vi "Main.vi"(11 "Module Admin":refnum<class "Delacor_lib_QMH_Module Admin.lvclass">) -> ()   [LabVIEW 2025, in "Scripting Server.lvlib"]
doc: "This template is based off of the Queued Message Handler design pattern and the Queued Message Handler project template that ships with LabVIEW.\n\nThe main difference is that the queue is private to this module and communication between modules is performed via Broadcast and Request events.\n\nRequest events are wrapped in public API methods and are handled in the Event Handling Loop (EHL) of this VI. Any module can register for Broadcast events sent by this module. The EHL generates messages based on user interface actions.\n\nThe Message Handling Loop (MHL) processes messages generated by the EHL, or by other messages. The messages are string values, so new messages can be added easily to the Message Cases case structure in the MHL. Each message cluster can also provide an optional value for Message Data, which is a variant that can be converted to whatever message-specific data is required.\n_____\nBased on DQMH Dev Tools: Project Template 7.1.0.1503."
uses:
  Scripting Server.lvlib
  <vilib>/Delacor/Delacor QMH/Libraries/Message Queue_class/Delacor_lib_QMH_Message Queue.lvclass/Delacor_lib_QMH_Message Queue.ctl
  <vilib>/Delacor/Delacor QMH/Libraries/Module Admin_class/Delacor_lib_QMH_Module Admin.lvclass/Delacor_lib_QMH_Module Admin.ctl
  <vilib>/Delacor/Delacor QMH/Libraries/Message Queue_class/Delacor_lib_QMH_Message Queue.lvclass
  Module Data--cluster.ctl
  <vilib>/Utility/miscctls.llb/LVPointTypeDef.ctl
  <vilib>/Delacor/Delacor QMH/Libraries/Message Queue_class/Delacor_lib_QMH_Enqueue Message (Single).vi
  Stop Argument--cluster.ctl
  <vilib>/Delacor/Delacor QMH/Libraries/Module Admin_class/Delacor_lib_QMH_Module Admin.lvclass
  New VI (Reply Payload)--cluster.ctl
  New VI Argument--cluster.ctl
  Add Object Argument--cluster.ctl
  Add Object (Reply Payload)--cluster.ctl
  Connect Objects (Reply Payload)--cluster.ctl
  Connect Objects Argument--cluster.ctl
  Get Object Terminals (Reply Payload)--cluster.ctl
  Get Object Terminals Argument--cluster.ctl
  get vi error list (Reply Payload)--cluster.ctl
  get vi error list Argument--cluster.ctl
  Cleanup VI (Reply Payload)--cluster.ctl
  Cleanup VI Argument--cluster.ctl
  create_control (Reply Payload)--cluster.ctl
  create_control Argument--cluster.ctl
  Run VI (Reply Payload)--cluster.ctl
  Run VI Argument--cluster.ctl
  add_to_selection (Reply Payload)--cluster.ctl
  add_to_selection Argument--cluster.ctl
  clear_selection_list (Reply Payload)--cluster.ctl
  clear_selection_list Argument--cluster.ctl
  remove_from_selection (Reply Payload)--cluster.ctl
  remove_from_selection Argument--cluster.ctl
  enclose_selection (Reply Payload)--cluster.ctl
  enclose_selection Argument--cluster.ctl
  rename_object (Reply Payload)--cluster.ctl
  rename_object Argument--cluster.ctl
  set_value (Reply Payload)--cluster.ctl
  set_value Argument--cluster.ctl
  delete_object (Reply Payload)--cluster.ctl
  delete_object Argument--cluster.ctl
  save_vi (Reply Payload)--cluster.ctl
  save_vi Argument--cluster.ctl
  get_structure_diagram (Reply Payload)--cluster.ctl
  get_structure_diagram Argument--cluster.ctl
  add_subvi (Reply Payload)--cluster.ctl
  add_subvi Argument--cluster.ctl
  connect_to_pane (Reply Payload)--cluster.ctl
  connect_to_pane Argument--cluster.ctl
  get_object_help (Reply Payload)--cluster.ctl
  get_object_help Argument--cluster.ctl
  get_loop_conditional_terminal (Reply Payload)--cluster.ctl
  get_loop_conditional_terminal Argument--cluster.ctl
  show_conditional_terminal (Reply Payload)--cluster.ctl
  show_conditional_terminal Argument--cluster.ctl
  get_loop_iteration_terminal (Reply Payload)--cluster.ctl
  get_loop_iteration_terminal Argument--cluster.ctl
  Config Data.ctl
  Read Config Data Argument--cluster.ctl
  get_allowed_paths (Reply Payload)--cluster.ctl
  get_allowed_paths Argument--cluster.ctl
  create_project (Reply Payload)--cluster.ctl
  create_project Argument--cluster.ctl
  Set Allowed Paths Argument--cluster.ctl
panel:
  in  "Ring 2":i32(ring)=2125 items=[".NET Container"=2125, ".NET Refnum"=3441, "2D Picture"=3508, "3D Picture"=23776, "Absolute Value"=1054, "Accept TLS"=1732, "Access Rights"=1412, "ActiveX Container"=2072, "Add"=1050, "Add (with error terminals)"=3915, "Add Array Elements"=1903, "Add Entropy"=1738, "Add Private Key To TLS Configuration"=1735, "Add Trusted Certificate To TLS Configuration"=1736, "Agitator"=3831, "AllSpoll"=1960, "Always Copy"=2400, "And"=1061, "And Array Elements"=1911, "Append True/False String"=1511, "Application Refnum"=3412, "Array (block diagram constant)"=2070, "Array (classic)"=3300, "Array (modern)"=21608, "Array Interface Control"=23777, "Array Max & Min"=1907, "Array of Strings to Path"=1422, "Array Size"=1809, "Array Subset"=2044, "Array To Cluster"=1168, "Array To Spreadsheet String"=1540, "ArrayMemInfo"=2412, "Assert Structural Type Match"=2416, "Assert Structural Type Mismatch"=2464, "Atmospheric Tank (classic)"=3070, "Atmospheric Tank (modern)"=21751, "Automation Close"=8001, "Automation Open"=8000, "Automation Refnum"=3410, "Avogadro Constant (1/mol)"=23520, "Base 10 Logarithm Of e"=23512, "Bin #1"=3073, "Bin #2"=21755, "Bitpack to Array"=3135, "Bluetooth Close Connection"=9148, "Bluetooth Create Listener"=9151, "Bluetooth Discover"=9152, "Bluetooth Network Connection Refnum"=3468, "Bluetooth Open Connection"=9153, "Bluetooth Read"=9149, "Bluetooth Wait On Listener"=9147, "Bluetooth Write"=9150, "Boolean Array To Number"=1815, "Boolean To (0,1)"=1167, "Build Array"=2041, "Build Cluster Array"=2047, "Build Map"=2463, "Build Matrix"=8500, "Build Path"=1419, "Build Set"=2462, "Build Waveform"=2066, "Bundle"=2049, "Bundle By Name"=2057, "Byte Array To String"=1609, "Byte Array To UTF-8 String"=1651, "Byte Stream File Refnum"=3408, "Call By Reference"=3901, "Call Chain"=1999, "Call Library Function Node"=2062, "Call MATLAB Function"=24210, "Call Parent Class Method"=2354, "CAN Channel (block diagram constant)"=2124, "CAN Channel (classic)"=3340, "CAN Channel (modern)"=21817, "CAN Channel (system)"=21966, "CAN Interface (block diagram constant)"=2123, "CAN Interface (classic)"=3339, "CAN Interface (modern)"=21815, "CAN Interface (system)"=21964, "CAN Task (block diagram constant)"=3471, "CAN Task (classic)"=3470, "CAN Task (modern)"=21789, "CAN Task (system)"=21963, "Cancel Button (modern)"=21739, "Cancel Button (system)"=3131, "Cancel Notification"=9107, "Carriage Return Constant"=23500, "Case Structure"=2001, "Cast Unit Bases"=1079, "Check Valve"=3833, "Checkbox (classic)"=3117, "CheckBox (modern)"=21924, "Checkbox (system)"=3132, "Class Specifier Constant"=2094, "Classic Color Box"=3013, "Classic Color Ramp"=3022, "Classic Horizontal Slide Switch"=3114, "Classic Vertical Slide"=3004, "Clear Fixed-Point Overflow Status"=5562, "Close File"=8052, "Close File (deprecated)"=1405, "Close MATLAB Session"=24209, "Close Python Session"=24207, "Close Reference"=8011, "Close TLS Configuration"=1741, "Close Variable Connection"=23783, "Closure Structure"=2372, "Cluster (classic)"=3400, "Cluster (modern)"=21607, "Cluster Constant"=2071, "Cluster To Array"=1169, "Code Interface Node"=2050, "Coerce To Type"=2402, "Collection Size"=2450, "Color Box Constant"=2120, "Color Box Thin Border"=2905, "Colored Rectangle (broken?)"=3625, "Combo Box (classic)"=3304, "Combo Box (modern)"=21604, "Combo Box (system)"=21917, "Combo Box Constant"=2088, "Complex Conjugate"=1048, "Complex To Polar"=1045, "Complex To Re/Im"=1044, "Compound Arithmetic"=2200, "Compressor"=3832, "Concatenate Strings"=2040, "Conditional Disable Structure"=2064, "Constructor Node"=3904, "Control & Simulation Loop"=2099, "Control Help Window"=1353, "Control Online Help"=1355, "Control Refnum"=3419, "Convert Unit"=2059, "Conveyer"=3827, "Copy"=8053, "Copy (deprecated)"=1416, "Cosecant"=1204, "Cosine"=1201, "Cotangent"=1205, "CPU Information"=24130, "Create Folder"=8055, "Create Network Stream Endpoint"=23793, "Create Network Stream Reader Endpoint"=23811, "Create Network Stream Writer Endpoint"=23810, "Create Stream"=23796, "Create Unique Network Stream Endpoint"=23795, "Create Unique Network Stream Reader Endpoint"=23807, "Create Unique Network Stream Writer Endpoint"=23806, "Create User Event"=2073, "Current Processor ID"=24131, "Current VI's Menubar"=9000, "Current VI's Path"=1426, "DAQmx Analog Trigger Source (block diagram constant)"=2119, "DAQmx Analog Trigger Source (classic)"=3336, "DAQmx Analog Trigger Source (modern)"=21774, "DAQmx Analog Trigger Source (system)"=21951, "DAQmx Device Name (block diagram constant)"=2093, "DAQmx Device Name (classic)"=3318, "DAQmx Device Name (modern)"=21773, "DAQmx Device Name (system)"=21950, "DAQmx Global Channel (block diagram constant)"=3430, "DAQmx Global Channel (classic)"=3443, "DAQmx Global Channel (modern)"=21770, "DAQmx Global Channel (system)"=21957, "DAQmx Physical Channel (block diagram constant)"=2118, "DAQmx Physical Channel (classic)"=3335, "DAQmx Physical Channel (modern)"=21777, "DAQmx Physical Channel (system)"=21954, "DAQmx Scale Name (block diagram constant)"=2116, "DAQmx Scale Name (classic)"=3317, "DAQmx Scale Name (modern)"=21775, "DAQmx Scale Name (system)"=21952, "DAQmx Switch (block diagram constant)"=2121, "DAQmx Switch (classic)"=3337, "DAQmx Switch (modern)"=21776, "DAQmx Switch (system)"=21953, "DAQmx Task Name (block diagram constant)"=3434, "DAQmx Task Name (classic)"=3442, "DAQmx Task Name (modern)"=21778, "DAQmx Task Name (system)"=21959, "DAQmx Terminal (block diagram constant)"=2117, "DAQmx Terminal (classic)"=3319, "DAQmx Terminal (modern)"=21781, "DAQmx Terminal (system)"=21955, "Data Cache Size"=24132, "Data Log File Refnum"=3402, "Data Value Reference"=3476, "Data Value Reference Constant"=24134, "DataSocket Close"=1085, "DataSocket Open"=1084, "DataSocket Read"=1086, "DataSocket Refnum"=3417, "DataSocket Write"=1087, "Date/Time To Seconds"=1308, "Decimal Digit?"=1119, "Decimal String To Number"=1184, "Decimate 1D Array"=2046, "DecomposeLockDataValRef"=2406, "DecomposeVariant"=2404, "Decrement"=1058, "Default Directory"=1427, "Delete"=8056, "Delete (deprecated)"=1417, "Delete Data Value Reference"=2409, "Delete From Array"=3912, "Delete Menu Items"=9004, "Delete Variant Attribute"=8206, "Delete Waveform Attribute"=8209, "Deny Access"=8057, "Dequeue Element"=9113, "Destroy Stream Endpoint"=23794, "Destroy User Event"=2075, "DevClear"=1961, "DevClearList"=1962, "Device Control/Status"=1433, "Device Refnum"=3405, "Diagram Disable Structure"=2054, "Dial (classic)"=3050, "Dial (modern)"=21732, "Digital Data (classic)"=3210, "Digital Data (modern)"=21216, "Digital Waveform Graph (classic)"=3511, "Digital Waveform Graph (modern)"=21718, "Direct Variable Read"=23785, "Direct Variable Write"=23788, "Divide"=1053, "Divide (with error terminals)"=3918, "Dlg Horiz Scrollbar"=21905, "Dlg Mac Group Box"=32514, "Dlg Numeric #1"=2100, "Dlg Numeric #2"=3006, "Dlg String"=2110, "Dlg Vert Scrollbar"=21906, "Down Arrow"=3824, "Down Bow Valve (flat)"=3707, "Down Bow Valve (outline)"=3807, "Down Bow Valve (shaded)"=21767, "Down Rect Valve (flat)"=3706, "Down Rect Valve (outline)"=3806, "Down Rect Valve (shaded)"=21766, "Down Tee (flat)"=3818, "Down Tee (shaded)"=3718, "Dynamic FPGA Interface Cast"=5690, "Eased Corner Rectangle"=32513, "Element of Set?"=2454, "Elementary Charge (C)"=23517, "Empty Array?"=23063, "Empty Collection?"=2451, "Empty Path Constant"=23523, "Empty String Constant"=23503, "Empty String/Path?"=1112, "Enable Menu Tracking"=9002, "EnableLocal"=1963, "EnableRemote"=1964, "End of Line Constant"=23525, "Enqueue Element"=9111, "Enqueue Element At Opposite End"=9129, "Enum (classic)"=3023, "Enum (modern)"=21605, "Enum (system)"=3062, "Enum Constant"=2090, "EOF"=1410, "Equal To 0?"=1113, "Equal?"=1102, "Error Ring Constant"=2039, "Event Callback Refnum"=3435, "Event Data Node"=2102, "Event Structure"=2052, "Exchanger"=3828, "Exclusive Or"=1063, "Exponential"=1211, "Exponential (Arg) -1"=1222, "Expression Node"=2201, "False Constant"=2006, "Feedback Node"=2353, "FieldPoint IO Point (block diagram constant)"=3440, "FieldPoint IO Point (classic)"=3439, "FieldPoint IO Point (modern)"=21784, "FIFO Refnum"=3474, "File Dialog"=8058, "File Dialog (deprecated)"=8081, "File Path Control (classic)"=3203, "File Path Control (modern)"=21730, "File Path Control (system)"=21922, "File Path Indicator (classic)"=3204, "File Path Indicator (modern)"=21731, "File/Directory Info"=8082, "File/Directory Info (deprecated)"=1413, "FindLstn"=1965, "FindRQS"=1966, "First Call?"=1083, "Fixed-Point Overflow?"=5565, "Fixed-Point to Integer Cast"=5566, "Flat Box"=3602, "Flat Circle"=3605, "Flat Down Triangle"=3623, "Flat Frame"=3608, "Flat Left Triangle"=3620, "Flat Right Triangle"=3621, "Flat Round Button"=3102, "Flat Rounded Box"=3611, "Flat Sequence Structure"=2069, "Flat Square Button"=3103, "Flat Up Triangle"=3622, "Flatten To JSON"=24201, "Flatten To String"=1164, "Flatten To XML"=8402, "Flattened String To Variant"=8202, "Floating Point Equal?"=23064, "Flush Event Queue"=2135, "Flush File"=8059, "Flush File (deprecated)"=1406, "Flush Queue"=9114, "Flush Stream"=23808, "For Loop"=2002, "Fork"=2194, "Format Date/Time String"=8100, "Format Into File"=2083, "Format Into String"=2081, "Format Value"=1512, "Formula Node"=2004, "FPGA Refnum to Session"=2322, "Fract/Exp String To Number"=1187, "Framed Color Box (classic)"=3008, "Framed Color Box (modern)"=21019, "Free Label"=2321, "Furnace"=3829, "Gauge (classic)"=3040, "Gauge (modern)"=21009, "Gauge for Simon"=32600, "Generate Front Panel Activity"=1329, "Generate Occurrence"=1700, "Generate User Event"=2074, "Generate User-Defined Trace Event"=2250, "Get Control Values by Index"=24204, "Get Datalog Position"=8061, "Get Date/Time In Seconds"=1303, "Get Date/Time String"=1600, "Get Drag Drop Data"=9154, "Get File Position"=8062, "Get File Size"=8063, "Get Fixed-Point Components"=11163, "Get Help Window Status"=1354, "Get Matrix Diagonal"=8501, "Get Matrix Elements"=8502, "Get Menu Item Info"=9005, "Get Menu Selection"=9001, "Get Menu Short Cut Info"=9007, "Get Notifier Status"=9103, "Get Number of Records"=8064, "Get Permissions"=8065, "Get Queue Status"=9110, "Get Submatrix"=8503, "Get Type and Creator"=8066, "Get Variant Attribute"=8205, "Get Volume Info"=8067, "Get Waveform Attribute"=8208, "Get Waveform Components"=2067, "Global Variable"=2060, "GPIB Clear"=1954, "GPIB Initialization"=1957, "GPIB Misc"=1956, "GPIB Read"=1951, "GPIB Serial Poll"=1955, "GPIB Status"=1959, "GPIB Trigger"=1953, "GPIB Wait"=1958, "GPIB Write"=1950, "Gravitational Constant (N m2/kg2)"=23519, "Greater Or Equal To 0?"=1114, "Greater Or Equal?"=1103, "Greater Than 0?"=1117, "Greater?"=1110, "Handle Peek"=1604, "Handle Poke"=1605, "Hex Digit?"=1123, "Hexadecimal String To Number"=1185, "Hopper #1"=21754, "Hopper #2"=3072, "Horiz Line"=3821, "Horiz Pipe (flat)"=3810, "Horiz Pipe (shaded)"=3710, "Horizontal Button Box"=3636, "Horizontal Fill Slide (classic)"=3012, "Horizontal Fill Slide (modern)"=21100, "Horizontal Gradient Oval"=32502, "Horizontal Gradient Rectangle"=32504, "Horizontal Gradient Rounded Rectangle"=32507, "Horizontal Graduated Bar"=21106, "Horizontal Pointer Slide (classic)"=3011, "Horizontal Pointer Slide (modern)"=21101, "Horizontal Pointer Slide (system)"=21902, "Horizontal Progress Bar (modern)"=21102, "Horizontal Progress Bar (system)"=21910, "Horizontal Scrollbar"=21110, "Horizontal Slide (classic)"=3010, "Horizontal Slide (system)"=21904, "Horizontal Smooth Box"=3633, "Horizontal Splitter Bar"=21861, "Horizontal Splitter Bar (Classic)"=21863, "Horizontal Splitter Bar (NXG Style)"=21867, "Horizontal Splitter Bar (System)"=21865, "Horizontal Switch"=3108, "Horizontal Tank"=3071, "Horizontal Toggle Switch (classic)"=3110, "Horizontal Toggle Switch (modern)"=21700, "Hyperbolic Cosecant"=23053, "Hyperbolic Cosine"=1215, "Hyperbolic Cotangent"=23055, "Hyperbolic Secant"=23054, "Hyperbolic Sine"=1214, "Hyperbolic Tangent"=1216, "IMAQ Session"=3415, "Implies"=1080, "In Place Element Structure"=2360, "In Range and Coerce"=1127, "Include Fixed-Point Overflow Status"=5564, "Increment"=1057, "Index & Bundle Cluster Array"=2056, "Index Array"=2042, "Index String Array"=1531, "Initialize Array"=2053, "Inline C Node"=2104, "Insert Into Array"=3911, "Insert Into Map"=2456, "Insert Into Set"=2452, "Insert Menu Items"=9003, "Integer to Fixed-Point Cast"=5567, "Intensity Chart (classic)"=3509, "Intensity Chart (modern)"=21719, "Intensity Graph (classic)"=3510, "Intensity Graph (modern)"=21720, "Interleave 1D Arrays"=2045, "Interpolate 1D Array"=1905, "Inverse Cosecant"=23050, "Inverse Cosine"=1207, "Inverse Cotangent"=23052, "Inverse Hyperbolic Cosecant"=23056, "Inverse Hyperbolic Cosine"=1218, "Inverse Hyperbolic Cotangent"=23058, "Inverse Hyperbolic Secant"=23057, "Inverse Hyperbolic Sine"=1217, "Inverse Hyperbolic Tangent"=1219, "Inverse Secant"=23051, "Inverse Sine"=1206, "Inverse Tangent"=1208, "Inverse Tangent (2 Input)"=1228, "Invoke Node"=3900, "IP To String"=1710, "IrDA Close Connection"=9144, "IrDA Create Listener"=9140, "IrDA Discover"=9141, "IrDA Network Connection Refnum"=3450, "IrDA Open Connection"=9142, "IrDA Read"=9145, "IrDA Wait On Listener"=9143, "IrDA Write"=9146, "IsDebuggingActive"=2403, "IVI Delete Session"=8103, "IVI Logical Name (block diagram constant)"=3420, "IVI Logical Name (classic)"=3414, "IVI Logical Name (modern)"=21736, "IVI New Session"=8102, "Join"=2195, "Join Numbers"=1171, "Junction"=2197, "Knob (classic)"=3005, "Knob (modern)"=21000, "Label (modern)"=21960, "Label (system)"=21961, "Labeled Oblong Button"=3125, "Labeled Rectangular Button"=3124, "Labeled Round Button"=3122, "Labeled Square Button"=3123, "LabVIEW Object"=3457, "Leak Variant Value Reference"=2410, "LED Button"=3116, "Left Arrow"=3826, "Left Bow Valve (flat)"=3701, "Left Bow Valve (outline)"=3801, "Left Bow Valve (shaded)"=21761, "Left Down Elbow (flat)"=3811, "Left Down Elbow (shaded)"=3711, "Left Pump (flat)"=3813, "Left Pump (shaded)"=3713, "Left Rect Valve (flat)"=3700, "Left Rect Valve (outline)"=3800, "Left Rect Valve (shaded)"=21760, "Left Tee (flat)"=3809, "Left Tee (shaded)"=3709, "Left Up Elbow (flat)"=3808, "Left Up Elbow (shaded)"=3708, "Less Or Equal To 0?"=1115, "Less Or Equal?"=1104, "Less Than 0?"=1118, "Less?"=1111, "Lexical Class"=1126, "Line (chiseled, system)"=3632, "Line (chiseled, thick)"=3630, "Line (chiseled, thin)"=3627, "Line (thick)"=3629, "Line (thin)"=3626, "Line Feed Constant"=23501, "Line with Arrow (thick)"=3631, "Line with Arrow (thin)"=3628, "List Directory"=1418, "List Folder"=8083, "Listbox (classic)"=21806, "Listbox (modern)"=21792, "Listbox (system)"=21805, "Listbox Symbol Ring Constant"=2038, "Load Certificates Into Memory"=1734, "Load Private Key Into Memory"=1733, "Local Variable"=2061, "Lock Range"=1411, "Logarithm Base 10"=1210, "Logarithm Base 2"=1225, "Logarithm Base X"=1224, "Logical Shift"=1081, "Look In Map"=2458, "Lookup Channel Probe"=9155, "Lossy Enqueue Element"=9130, "Lowered Box (thick)"=3635, "Lowered Rounded Box"=3638, "Machine Epsilon"=23528, "Make TLS Configuration Immutable"=1737, "MakeAddr"=1967, "Mantissa & Exponent"=1150, "Map"=3488, "Map Constant"=2461, "Match First String"=1532, "Match Pattern"=1535, "Match True/False String"=1533, "MathScript Call By Reference"=3906, "MathScript Node"=2357, "MATLAB script"=9020, "MATLAB Session Refnum"=3490, "Matrix Size"=8507, "Max & Min"=1108, "Menu Refnum"=3413, "Menu Ring (classic)"=3018, "Menu Ring (modern)"=21600, "Menu-Popup Ring"=3017, "Merge Errors"=2147, "Merge Signals"=2350, "Meter (classic)"=3030, "Meter (modern)"=21008, "Mixed Checkbox (system)"=21333, "Mixed Signal Graph"=21721, "Molar Gas Constant (J/(mol K))"=23522, "Motion Resource (block diagram constant)"=3449, "Motion Resource (classic)"=3448, "Motion Resource (modern)"=21787, "Motor (flat)"=3820, "Motor (shaded)"=3720, "Move"=8068, "Move (deprecated)"=1415, "Multi-Segment Pipe"=23780, "Multicolumn Listbox (classic)"=21799, "Multicolumn Listbox (modern)"=21791, "Multicolumn Listbox (system)"=21798, "Multiply"=1052, "Multiply (with error terminals)"=3917, "Multiply Array Elements"=1904, "Multirate Structure"=2199, "Natural Logarithm"=1209, "Natural Logarithm (Arg +1)"=1221, "Natural Logarithm Base"=23510, "Natural Logarithm Of 10"=23513, "Natural Logarithm Of 2"=23514, "Natural Logarithm Of Pi"=23508, "Negate"=1069, "Negative Infinity"=23509, "New Data Value Reference"=2408, "New Directory"=1402, "New File"=1404, "New TLS Configuration"=1730, "New VI"=8014, "New VI Object"=8015, "Not"=1064, "Not A Number/Path/Refnum?"=1128, "Not A Path Constant"=23524, "Not a Refnum Constant"=23526, "Not a Shared Variable"=23527, "Not And"=1071, "Not Equal To 0?"=1116, "Not Equal?"=1105, "Not Exclusive Or"=1073, "Not Or"=1072, "Notifier Refnum"=3423, "Number of Cache Levels"=24133, "Number To Boolean Array"=1814, "Number To Decimal String"=1180, "Number To Engineering String"=1183, "Number To Exponential String"=1505, "Number To Fractional String"=1506, "Number To Hexadecimal String"=1181, "Number To Octal String"=1182, "Numeric Constant"=2005, "Numeric Control (classic)"=3000, "Numeric Control (modern)"=21003, "Numeric Control (system)"=21919, "Numeric Indicator (classic)"=3001, "Numeric Indicator (modern)"=21004, "Obtain Notifier"=9101, "Obtain Queue"=9108, "Occurrence Refnum"=3406, "Octal Digit?"=1129, "Octal String To Number"=1186, "OK Button (modern)"=21738, "OK Button (system)"=3130, "Old VISA Open"=1921, "OLE Variant"=3150, "One Button Dialog"=1340, "Open and Verify Variable Connection"=23790, "Open Application Reference"=8012, "Open Device"=1430, "Open Dynamic Bitfile Reference"=5691, "Open File"=1403, "Open MATLAB Session"=24208, "Open Python Session"=24206, "Open Tank (flat classic)"=21752, "Open Tank (shaded classic)"=3074, "Open Variable Connection"=23779, "Open Variable Connection in Background"=23791, "Open VI Object Reference"=8013, "Open VI Reference"=8010, "Open/Create/Replace Datalog"=8054, "Open/Create/Replace File"=8050, "Or"=1062, "Or Array Elements"=1910, "Oval with Shadow"=32509, "Package Matrix"=23001, "PassControl"=1968, "Path Constant"=2009, "Path to Array of Strings"=1423, "Path To String"=1077, "Path Type"=1421, "Pi"=23504, "Pi Divided By 2"=23506, "Pi Multiplied By 2"=23505, "Pick Line"=1510, "Pict Ring (classic)"=3015, "Pict Ring (modern)"=21602, "Pict Ring (system)"=21925, "PixMap"=3505, "PixMap (warning: dangerous)"=3507, "Planck's Constant (J/Hz)"=23516, "Platform Flat Square Button"=3134, "Plug-In Control"=21820, "Polar To Complex"=1047, "Polar To Re/Im"=23061, "Positive Infinity"=23515, "Power Of 10"=1212, "Power Of 2"=1223, "Power Of X"=1213, "PPoll"=1969, "PPollConfig"=1970, "PPollUnconfig"=1971, "Preallocated Read from Binary File"=24135, "Preserve Run-Time Class"=8018, "Pressure Tank (flat)"=3075, "Pressure Tank (shaded)"=21753, "Preview Queue Element"=9112, "Printable?"=1124, "Property Node"=1920, "Pulldown Menu Ring"=3061, "Push Button"=21001, "Python Node"=24205, "Python Session Refnum"=3486, "Queue Refnum"=3424, "Quit LabVIEW"=1352, "Quotient & Remainder"=1056, "Race Structure"=2371, "Radio Button (system)"=3133, "Radio Buttons (classic)"=22003, "Radio Buttons (modern)"=22001, "Radio Buttons (system)"=22002, "Raised Box (classic)"=3600, "Raised Box (modern)"=3637, "Raised Circle"=3603, "Raised Down Triangle"=3615, "Raised Frame"=3606, "Raised Left Triangle"=3612, "Raised Right Triangle"=3613, "Raised Rounded Box"=3609, "Raised Up Triangle"=3614, "Random Number (0-1)"=1070, "RcvRespMsg"=1972, "Re-accept TLS"=1739, "Re/Im To Complex"=1046, "Re/Im To Polar"=23060, "Read Datalog"=8069, "Read Device"=1432, "Read File"=1407, "Read from Binary File"=8051, "Read from Text File"=8070, "Read Map Max & Min Keys"=2459, "Read Multiple Elements from Stream"=23803, "Read Set Max & Min"=2455, "Read Single Element from Stream"=23797, "Read Variable"=23781, "Read Variable with Timeout"=23786, "ReadStatus"=1973, "Receive"=1974, "ReceiveSetup"=1975, "Recessed Box"=3601, "Recessed Circle"=3604, "Recessed Down Triangle"=3619, "Recessed Frame (modern)"=3607, "Recessed Frame (system)"=3624, "Recessed Left Triangle"=3616, "Recessed Menu Ring"=3019, "Recessed Right Triangle"=3617, "Recessed Rounded Box"=3610, "Recessed Up Triangle"=3618, "Reciprocal"=1059, "Reciprocal Of e"=23511, "Reciprocal Of Pi"=23507, "RecomposeUnlockDataValRef (warning: dangerous)"=2407, "RecomposeVariant (warning: dangerous)"=2405, "Rectangular Stop Button"=3128, "Refnum to Path"=1424, "Refnum to Session"=2306, "Region"=2196, "Register Event Callback"=2078, "Register For Events"=2065, "Register Session"=2319, "Release Notifier"=9102, "Release Queue"=9109, "Remove Fixed-Point Overflow Status"=5563, "Remove From Map"=2457, "Remove From Set"=2453, "Replace Array Subset"=3910, "Replace Substring"=3913, "Request Deallocation"=1610, "ResetSys"=1976, "Reshape Array"=2055, "Resize Matrix"=8508, "Resource Index"=1088, "Reverse 1D Array"=1900, "Reverse String"=1537, "Right Arrow"=3825, "Right Bow Valve (flat)"=3705, "Right Bow Valve (outline)"=3805, "Right Bow Valve (shaded)"=21765, "Right Down Elbow (flat)"=3817, "Right Down Elbow (shaded)"=3717, "Right Pump (flat)"=3819, "Right Pump (shaded)"=3719, "Right Rect Valve (flat)"=3704, "Right Rect Valve (outline)"=3804, "Right Rect Valve (shaded)"=21764, "Right Tee (flat)"=3815, "Right Tee (shaded)"=3715, "Right Up Elbow (flat)"=3814, "Right Up Elbow (shaded)"=3714, "Rocker"=21002, "Rotary Feeder"=3830, "Rotate"=1082, "Rotate 1D Array"=1906, "Rotate Left With Carry"=1606, "Rotate Right With Carry"=1607, "Rotate String"=1536, "Round Button"=3100, "Round LED (classic)"=3120, "Round LED (modern)"=21012, "Round Light"=3104, "Round Push Button"=3118, "Round Push Button (profile)"=3112, "Round Radio Button"=3106, "Round Stop Button"=3127, "Round To Nearest"=1055, "Round Toward +Infinity"=1076, "Round Toward -Infinity"=1075, "Rounded Rectangle with Shadow"=32508, "RT FIFO Create"=24000, "RT FIFO Delete"=24003, "RT FIFO Read"=24001, "RT FIFO Write"=24002, "Rydberg Constant (1/m)"=23521, "Scale By Power Of 2"=1074, "Scan From File"=2082, "Scan From String"=2080, "Scan String For Tokens"=8101, "Scan Value"=1534, "Scanned Variable Read"=23784, "Scanned Variable Write"=23787, "Search 1D Array"=1901, "Search and Replace String"=3914, "Search Variable Container"=23802, "Search/Split String"=1538, "Secant"=1203, "Seconds To Date/Time"=1309, "Seek"=1409, "Select"=1516, "Send"=1977, "Send Notification"=9104, "SendCmds"=1978, "SendDataBytes"=1979, "SendIFC"=1980, "SendList"=1981, "SendLLO"=1982, "SendSetup"=1983, "Session to Refnum"=2307, "Set"=3487, "Set Constant"=2460, "Set Control Values by Index"=24203, "Set Datalog Position"=8072, "Set File Position"=8073, "Set File Size"=8074, "Set Matrix Diagonal"=8504, "Set Matrix Elements"=8505, "Set Menu Item Info"=9006, "Set Number of Records"=8075, "Set Occurrence"=1702, "Set Permissions"=8076, "Set Submatrix"=8506, "Set Type and Creator"=8077, "Set Variant Attribute"=8204, "Set Waveform Attribute"=8207, "SetRWLS"=1984, "SetTimeOut"=1985, "Shared Variable"=23778, "Shared Variable Constant"=3473, "Shared Variable Control (classic)"=3472, "Shared Variable Control (modern)"=21814, "Shared Variable to String"=1831, "Sign"=1049, "Simple Horizontal Slide"=3003, "Simple Numeric"=2900, "Simple String"=2115, "Simple Vertical Slide"=3002, "Sinc"=1227, "Sine"=1200, "Sine & Cosine"=1220, "Size Handle"=1603, "Slide Switch"=21011, "Smoothed Oval"=32500, "Smoothed Rounded Rectangle"=32505, "Sort 1D Array"=1120, "Sort Array of String"=23065, "Speed Of Light In Vacuum (m/sec)"=23518, "Spin Control (system)"=21900, "Split 1D Array"=1908, "Split Button"=21020, "Split Number"=1170, "Split Signals"=2351, "Spreadsheet String To Array"=1539, "Square"=23059, "Square Button"=3101, "Square LED (classic)"=3121, "Square LED (modern)"=21013, "Square Light"=3105, "Square Push Button"=3119, "Square Push Button (profile)"=3113, "Square Radio Button"=3107, "Square Root"=1060, "Stacked Sequence Structure"=2000, "Start TLS"=1731, "State"=2198, "State Diagram"=2051, "Static VI Reference"=2084, "Stop"=1350, "Stop Button"=21230, "String Constant"=2007, "String Control (classic)"=3200, "String Control (modern)"=21701, "String Control (system)"=21920, "String Indicator (classic)"=3201, "String Indicator (modern)"=21702, "String Length"=1502, "String Subset"=1503, "String To Byte Array"=1608, "String To IP"=1711, "String To Path"=1078, "String to Shared Variable"=1830, "Strip Path"=1420, "SubPanel"=21810, "SubPanel (Classic)"=21811, "SubPanel (NXG Style)"=21824, "SubPanel (System)"=21823, "Subtract"=1051, "Subtract (with error terminals)"=3916, "Swap Bytes"=1162, "Swap Values"=2401, "Swap Vector Element"=1912, "Swap Words"=1163, "Tab Constant"=23502, "Tab Control (classic)"=3330, "Tab Control (modern)"=3332, "Tab Control (NXG Style)"=32700, "Tab Control (system)"=3331, "Table (classic)"=21796, "Table (modern)"=21790, "Table (system)"=21797, "Tag Attribute Ring"=2063, "Tangent"=1202, "Tank (classic)"=3020, "Tank (modern)"=21006, "Target Structure"=2370, "TCP Close Connection"=1713, "TCP Create Listener"=1717, "TCP Flattened Read"=1718, "TCP Flattened Write"=1719, "TCP Flex Read"=1720, "TCP Flex Write"=1721, "TCP Network Connection Refnum"=3407, "TCP Open Connection"=1715, "TCP Read"=1716, "TCP Wait On Listener"=1712, "TCP Write"=1714, "TDMS Advanced Asynchronous Read (Data Ref)"=2151, "TDMS Advanced Asynchronous Write (Data Ref)"=2150, "TDMS Close"=24113, "TDMS Configure Asynchronous Reads (Data Ref)"=2153, "TDMS Configure Asynchronous Writes (Data Ref)"=2152, "TDMS Defragment"=24119, "TDMS Delete Data"=2159, "TDMS File"=3477, "TDMS Flush"=24117, "TDMS Get Asynchronous Read Status (Data Ref)"=2155, "TDMS Get Asynchronous Write Status (Data Ref)"=2154, "TDMS Get Properties"=24115, "TDMS In Memory Close"=2157, "TDMS In Memory Open"=2156, "TDMS In Memory Read Bytes"=2158, "TDMS List Contents"=24116, "TDMS Open"=24112, "TDMS Read"=24111, "TDMS Refnum To File ID"=24120, "TDMS Set Properties"=24114, "TDMS Write"=24110, "TDMS Write IP"=24118, "Temporary Directory"=1435, "TestSRQ"=1986, "TestSys"=1987, "Text & Pict Ring (classic)"=3016, "Text & Pict Ring (modern)"=21603, "Text Button"=21015, "Text Ring (block diagram constant)"=2008, "Text Ring (classic)"=3014, "Text Ring (modern)"=21601, "Text Ring (system)"=3060, "Text to UTF-8"=23066, "Thermometer (classic)"=3021, "Thermometer (modern)"=21007, "Threshold 1D Array"=1909, "Tick Count (ms)"=1300, "Time Stamp (block diagram constant)"=2068, "Time Stamp Control (classic)"=5555, "Time Stamp Control (modern)"=21913, "Time Stamp Control (system)"=21967, "Time Stamp Indicator (classic)"=5556, "Time Stamp Indicator (modern)"=21914, "Timed Loop"=5570, "Timed Sequence"=5573, "TLS configuration"=3489, "TLS Connection?"=1740, "To Byte Integer"=1140, "To Double Precision Complex"=1152, "To Double Precision Float"=1147, "To Extended Precision Complex"=1154, "To Extended Precision Float"=1149, "To Fixed-Point"=5561, "To Long Integer"=1142, "To Lower Case"=1189, "To More Generic Class"=8017, "To More Specific Class"=8016, "To OLE Variant"=8002, "To Probe String"=2413, "To Quad Integer"=1155, "To Single Precision Complex"=1151, "To Single Precision Float"=1146, "To Time Stamp"=5560, "To Unsigned Byte Integer"=1143, "To Unsigned Long Integer"=1145, "To Unsigned Quad Integer"=1156, "To Unsigned Word Integer"=1144, "To Upper Case"=1188, "To Variant"=8201, "To Word Integer"=1141, "Traditional DAQ Channel (block diagram constant)"=2085, "Traditional DAQ Channel (classic)"=3320, "Traditional DAQ Channel (modern)"=21733, "Transpose 1D Array"=23068, "Transpose 2D Array"=1902, "Transpose Matrix"=8509, "Tree (classic)"=21819, "Tree (modern)"=21793, "Tree (system)"=21794, "Trigger"=1988, "TriggerList"=1989, "Two Button Dialog"=1341, "Type and Creator"=1434, "Type Cast"=1166, "Type Error"=2415, "Type Must Be Array"=2417, "Type Must Be Cluster"=2418, "Type Of"=2414, "Type Specialization Structure"=2373, "UDP Close"=1726, "UDP Multicast Open"=1727, "UDP Network Connection Refnum"=3418, "UDP Open"=1723, "UDP Read"=1724, "UDP Write"=1725, "Unbitpack from Array"=3136, "Unbundle"=2048, "Unbundle By Name"=2058, "Unflatten From JSON"=24202, "Unflatten From String"=1165, "Unflatten From XML"=8401, "Unleak Variant Value Reference"=2411, "Unpackage Matrix"=23000, "Unregister For Events"=2076, "Unregister Session"=2320, "Up Arrow"=3823, "Up Bow Valve (flat)"=3703, "Up Bow Valve (outline)"=3803, "Up Bow Valve (shaded)"=21763, "Up Rect Valve (flat)"=3702, "Up Rect Valve (outline)"=21762, "Up Rect Valve (shaded)"=3802, "Up Tee (flat)"=3812, "Up Tee (shaded)"=3712, "User Defined Refnum"=3428, "User Defined Refnum Tag (block diagram constant)"=3426, "User Defined Refnum Tag (classic)"=3429, "User Defined Refnum Tag (modern)"=21745, "User Defined Refnum Tag Flatten (classic)"=3454, "User Defined Refnum Tag Flatten (modern)"=21747, "User Defined Tag (block diagram constant)"=2114, "User Defined Tag (classic)"=3329, "User Defined Tag (modern)"=21749, "User Item"=3506, "UTF-8 String To Byte Array"=1650, "UTF-8 to Text"=23067, "Variable Class Specifier Constant"=2106, "Variable Name Constant"=3478, "Variant"=3310, "Variant To Data"=8003, "Variant To Flattened String"=8203, "Vert Line"=3822, "Vert Pipe (flat)"=3816, "Vert Pipe (shaded)"=3716, "Vert Rocker"=21740, "Vertical Fill Slide (classic)"=3009, "Vertical Fill Slide (modern)"=21014, "Vertical Gradient Oval"=32501, "Vertical Gradient Rectangle"=32503, "Vertical Gradient Rounded Rectangle"=32506, "Vertical Graduated Bar"=21107, "Vertical Pointer Slide (classic)"=3007, "Vertical Pointer Slide (modern)"=21017, "Vertical Pointer Slide (system)"=21901, "Vertical Progress Bar (modern)"=21104, "Vertical Progress Bar (system)"=21909, "Vertical Scrollbar"=21111, "Vertical Slide (system)"=21903, "Vertical Slide Switch (classic)"=3115, "Vertical Slide Switch (modern)"=21741, "Vertical Smooth Box"=3634, "Vertical Splitter Bar"=21860, "Vertical Splitter Bar (Classic)"=21862, "Vertical Splitter Bar (NXG Style)"=21866, "Vertical Splitter Bar (System)"=21864, "Vertical Switch"=3109, "Vertical Toggle Switch (classic)"=3111, "Vertical Toggle Switch (modern)"=21005, "VI Library"=1425, "VI Refnum"=3422, "VI Server Reference"=2091, "VISA Assert Interrupt Signal"=2309, "VISA Assert Trigger"=1929, "VISA Assert Utility Signal"=2310, "VISA Clear"=1927, "VISA Close"=1922, "VISA Disable Event"=1940, "VISA Discard Events"=1941, "VISA Enable Event"=1942, "VISA Find Resource"=1923, "VISA Flush I/O Buffer"=2302, "VISA GPIB Command"=2315, "VISA GPIB Control ATN"=2316, "VISA GPIB Control REN"=2304, "VISA GPIB Pass Control"=2317, "VISA GPIB Send IFC"=2318, "VISA In 16"=1930, "VISA In 32"=1944, "VISA In 64"=2140, "VISA In 8"=1936, "VISA Lock"=1993, "VISA Map Address"=1932, "VISA Map Trigger"=2311, "VISA Memory Allocation"=1997, "VISA Memory Allocation Ex"=2146, "VISA Memory Free"=1998, "VISA Move"=2303, "VISA Move In 16"=1948, "VISA Move In 32"=1991, "VISA Move In 64"=2144, "VISA Move In 8"=1946, "VISA Move Out 16"=1949, "VISA Move Out 32"=1992, "VISA Move Out 64"=2145, "VISA Move Out 8"=1947, "VISA Open"=2308, "VISA Out 16"=1931, "VISA Out 32"=1945, "VISA Out 64"=2141, "VISA Out 8"=1937, "VISA Peek 16"=1934, "VISA Peek 32"=1995, "VISA Peek 64"=2142, "VISA Peek 8"=1938, "VISA Poke 16"=1935, "VISA Poke 32"=1996, "VISA Poke 64"=2143, "VISA Poke 8"=1939, "VISA Read"=1925, "VISA Read STB"=1928, "VISA Read To File"=2313, "VISA Refnum to Session"=2300, "VISA Resource Name"=3421, "VISA resource name (classic)"=3409, "VISA resource name (modern)"=21737, "VISA Set I/O Buffer Size"=2301, "VISA Status Description"=1924, "VISA Unlock"=1994, "VISA Unmap Address"=1933, "VISA Unmap Trigger"=2312, "VISA USB Control In"=2086, "VISA USB Control Out"=2087, "VISA VXI Cmd or Query"=2305, "VISA Wait on Event"=1943, "VISA Write"=1926, "VISA Write From File"=2314, "Volume Info"=1414, "Wait (ms)"=1302, "Wait For Activity"=1722, "Wait For Front Panel Activity"=1328, "Wait for GPIB RQS"=1952, "Wait on Notification"=9105, "Wait on Notification from Multiple"=9106, "Wait on Notification from Multiple with Notifier History"=9132, "Wait on Notification with Notifier History"=9131, "Wait on Occurrence"=1701, "Wait Until Next ms Multiple"=1327, "WaitSRQ"=1990, "Waveform Chart"=21010, "Waveform Chart (classic)"=3501, "Waveform Chart (modern)"=21717, "Waveform Graph (classic)"=3504, "Waveform Graph (modern)"=21703, "While Loop #1"=2003, "While Loop #2"=2352, "White Space?"=1125, "Write Datalog"=8079, "Write Device"=1431, "Write File"=1408, "Write Multiple Elements to Stream"=23804, "Write Single Element to Stream"=23798, "Write to Binary File"=8078, "Write to Text File"=8080, "Write Variable"=23782, "Write Variable with Timeout"=23789, "XY Graph (classic)"=3500, "XY Graph (modern)"=21716, "Y-th Root of X"=23062]
  out "error out":errorcluster
  out "Status":string
  in  "Simulate MHL Error":bool
  in  "Simulate EHL Error":bool
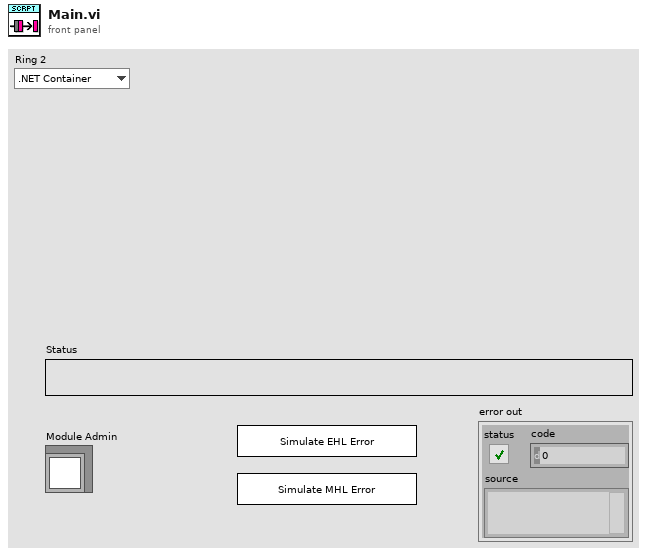
[diagram p1: front panel]
types:
  T1 = typedef "Scripting Server.lvlib/Request Events--cluster.ctl" = cluster{"Stop Module":refnum<user-event>, "Show Panel":refnum<user-event>, "Hide Panel":refnum<user-event>, "Get Module Execution Status":refnum<user-event>, "Show Diagram":refnum<user-event>, "New VI":refnum<user-event>, "Add Object":refnum<user-event>, "Connect Objects":refnum<user-event>, "Get Object Terminals":refnum<user-event>, "get vi error list":refnum<user-event>, "Cleanup VI":refnum<user-event>, "create_control":refnum<user-event>, "Run VI":refnum<user-event>, "add_to_selection":refnum<user-event>, "clear_selection_list":refnum<user-event>, "remove_from_selection":refnum<user-event>, "enclose_selection":refnum<user-event>, "rename_object":refnum<user-event>, "set_value":refnum<user-event>, "delete_object":refnum<user-event>, "save_vi":refnum<user-event>, "get_structure_diagram":refnum<user-event>, "add_subvi":refnum<user-event>, "connect_to_pane":refnum<user-event>, "get_object_help":refnum<user-event>, "get_loop_conditional_terminal":refnum<user-event>, "show_conditional_terminal":refnum<user-event>, "get_loop_iteration_terminal":refnum<user-event>, "Read Config Data":refnum<user-event>, "get_allowed_paths":refnum<user-event>, "create_project":refnum<user-event>, "Set Allowed Paths":refnum<user-event>}
  T2 = typedef "Scripting Server.lvlib/Module Data--cluster.ctl" = cluster{"Status":string, "Current ID":i32, "References":variant, "Config Data":T3}
  T3 = typedef "Scripting Server.lvlib/Config Data.ctl" = cluster{"Allowed Paths":string[]}
  T4 = enum32{"invalid lock state", "Not Locked", "Locked (No Password)", "Password-protected"}
  T5 = typedef "Scripting Server.lvlib/Stop Argument--cluster.ctl" = cluster{"Origin":string, "Exit via Stop Module Req?":bool, "Wait for Module to stop?":bool}
  T6 = typedef "Scripting Server.lvlib/New VI Argument--cluster.ctl" = cluster{"Open Frontpanel":bool, "Wait Notifier":refnum<notifier>, "wait for reply":bool}
  T7 = typedef "Scripting Server.lvlib/Add Object Argument--cluster.ctl" = cluster{"VI Reference":i32, "Object Name":string, "Wait Notifier":refnum<notifier>, "wait for reply":bool, "position_x":i32, "position_y":i32}
  T8 = typedef "Scripting Server.lvlib/Connect Objects Argument--cluster.ctl" = cluster{"vi reference":i32, "from object reference":i32, "to object reference":i32, "from object terminal index":i32, "to object terminal index":i32, "Wait Notifier":refnum<notifier>, "wait for reply":bool}
  T9 = typedef "Scripting Server.lvlib/Get Object Terminals Argument--cluster.ctl" = cluster{"object id":i32, "Wait Notifier":refnum<notifier>, "wait for reply":bool}
  T10 = typedef "Scripting Server.lvlib/get vi error list Argument--cluster.ctl" = cluster{"vi id":i32, "Wait Notifier":refnum<notifier>, "wait for reply":bool}
  T11 = typedef "Scripting Server.lvlib/Cleanup VI Argument--cluster.ctl" = cluster{"vi reference":i32, "Wait Notifier":refnum<notifier>, "wait for reply":bool}
  T12 = typedef "Scripting Server.lvlib/create_control Argument--cluster.ctl" = cluster{"Object ID":i32, "Terminal Index":i32, "Constant":bool, "Wait Notifier":refnum<notifier>, "wait for reply":bool, "Value":string}
  T13 = typedef "Scripting Server.lvlib/Run VI Argument--cluster.ctl" = cluster{"VI ID":i32, "open_frontpanel":bool, "Wait Notifier":refnum<notifier>, "wait for reply":bool}
  T14 = typedef "Scripting Server.lvlib/add_to_selection Argument--cluster.ctl" = cluster{"object_id":i32, "Wait Notifier":refnum<notifier>, "wait for reply":bool, "vi_id":i32}
  T15 = typedef "Scripting Server.lvlib/clear_selection_list Argument--cluster.ctl" = cluster{"Wait Notifier":refnum<notifier>, "wait for reply":bool, "vi_id":i32}
  T16 = typedef "Scripting Server.lvlib/remove_from_selection Argument--cluster.ctl" = cluster{"vi_id":i32, "object_id":i32, "Wait Notifier":refnum<notifier>, "wait for reply":bool}
  T17 = typedef "Scripting Server.lvlib/enclose_selection Argument--cluster.ctl" = cluster{"vi_id":i32, "structure_type":string, "Wait Notifier":refnum<notifier>, "wait for reply":bool}
  T18 = typedef "Scripting Server.lvlib/rename_object Argument--cluster.ctl" = cluster{"new_label_name":string, "label_visible":bool, "Wait Notifier":refnum<notifier>, "wait for reply":bool, "object_id":i32}
  T19 = typedef "Scripting Server.lvlib/set_value Argument--cluster.ctl" = cluster{"object_id":i32, "value":string, "Wait Notifier":refnum<notifier>, "wait for reply":bool}
  T20 = typedef "Scripting Server.lvlib/delete_object Argument--cluster.ctl" = cluster{"object_id":i32, "Wait Notifier":refnum<notifier>, "wait for reply":bool}
  T21 = typedef "Scripting Server.lvlib/save_vi Argument--cluster.ctl" = cluster{"vi_id":i32, "path":string, "Wait Notifier":refnum<notifier>, "wait for reply":bool}
  T22 = typedef "Scripting Server.lvlib/get_structure_diagram Argument--cluster.ctl" = cluster{"structure_id":i32, "index":i32, "Wait Notifier":refnum<notifier>, "wait for reply":bool}
  T23 = typedef "Scripting Server.lvlib/add_subvi Argument--cluster.ctl" = cluster{"diagram_id":i32, "subvi_path":string, "Wait Notifier":refnum<notifier>, "wait for reply":bool, "position_x":i32, "position_y":i32}
  T24 = typedef "Scripting Server.lvlib/connect_to_pane Argument--cluster.ctl" = cluster{"control_id":i32, "connector_pane_index":i32, "Wait Notifier":refnum<notifier>, "wait for reply":bool}
  T25 = typedef "Scripting Server.lvlib/get_object_help Argument--cluster.ctl" = cluster{"object_id":i32, "Wait Notifier":refnum<notifier>, "wait for reply":bool}
  T26 = typedef "Scripting Server.lvlib/get_loop_conditional_terminal Argument--cluster.ctl" = cluster{"loop_id":i32, "Wait Notifier":refnum<notifier>, "wait for reply":bool}
  T27 = typedef "Scripting Server.lvlib/show_conditional_terminal Argument--cluster.ctl" = cluster{"loop_id":i32, "show":bool, "Wait Notifier":refnum<notifier>, "wait for reply":bool}
  T28 = typedef "Scripting Server.lvlib/get_loop_iteration_terminal Argument--cluster.ctl" = cluster{"loop_id":i32, "Wait Notifier":refnum<notifier>, "wait for reply":bool}
  T29 = typedef "Scripting Server.lvlib/Read Config Data Argument--cluster.ctl" = cluster{"Boolean":bool}
  T30 = typedef "Scripting Server.lvlib/get_allowed_paths Argument--cluster.ctl" = cluster{"Wait Notifier":refnum<notifier>, "wait for reply":bool}
  T31 = typedef "Scripting Server.lvlib/create_project Argument--cluster.ctl" = cluster{"File Path":string, "Wait Notifier":refnum<notifier>, "wait for reply":bool}
  T32 = typedef "Scripting Server.lvlib/Set Allowed Paths Argument--cluster.ctl" = cluster{"Working Directory Folder Path":path[]}
  T33 = typedef "LVPointTypeDef.ctl" = cluster{"Horizontal":i16, "Vertical":i16}
  T34 = enum32{"Invalid", "Standard", "Closed", "Hidden", "Minimized", "Maximized"}
  T35 = typedef "Scripting Server.lvlib/New VI (Reply Payload)--cluster.ctl" = cluster{"VI Reference":i32, "Result":string, "error":errorcluster}
  T36 = typedef "Scripting Server.lvlib/Add Object (Reply Payload)--cluster.ctl" = cluster{"error":errorcluster, "Object ID":i32, "Result":string}
  T37 = typedef "Scripting Server.lvlib/Connect Objects (Reply Payload)--cluster.ctl" = cluster{"result":string, "error":errorcluster}
  T38 = typedef "Scripting Server.lvlib/Get Object Terminals (Reply Payload)--cluster.ctl" = cluster{"terminals description":string, "error":errorcluster}
  T39 = typedef "Scripting Server.lvlib/get vi error list (Reply Payload)--cluster.ctl" = cluster{"error list":string, "error":errorcluster}
  T40 = typedef "Scripting Server.lvlib/create_control (Reply Payload)--cluster.ctl" = cluster{"Object ID":i32, "error":errorcluster}
  T41 = typedef "Scripting Server.lvlib/Run VI (Reply Payload)--cluster.ctl" = cluster{"error":errorcluster}
  T42 = typedef "Scripting Server.lvlib/add_to_selection (Reply Payload)--cluster.ctl" = cluster{"Current Selection":i32[], "error":errorcluster}
  T43 = typedef "Scripting Server.lvlib/clear_selection_list (Reply Payload)--cluster.ctl" = cluster{"error":errorcluster}
  T44 = typedef "Scripting Server.lvlib/remove_from_selection (Reply Payload)--cluster.ctl" = cluster{"current_selection":i32[], "error":errorcluster}
  T45 = typedef "Scripting Server.lvlib/enclose_selection (Reply Payload)--cluster.ctl" = cluster{"object_id":i32, "error":errorcluster}
  T46 = typedef "Scripting Server.lvlib/rename_object (Reply Payload)--cluster.ctl" = cluster{"error":errorcluster}
  T47 = typedef "Scripting Server.lvlib/set_value (Reply Payload)--cluster.ctl" = cluster{"error":errorcluster}
  T48 = typedef "Scripting Server.lvlib/delete_object (Reply Payload)--cluster.ctl" = cluster{"error":errorcluster}
  T49 = typedef "Scripting Server.lvlib/save_vi (Reply Payload)--cluster.ctl" = cluster{"path_out":string, "error":errorcluster}
  T50 = typedef "Scripting Server.lvlib/get_structure_diagram (Reply Payload)--cluster.ctl" = cluster{"diagram_id":i32, "error":errorcluster}
  T51 = typedef "Scripting Server.lvlib/add_subvi (Reply Payload)--cluster.ctl" = cluster{"subvi_id":i32, "error":errorcluster}
  T52 = typedef "Scripting Server.lvlib/connect_to_pane (Reply Payload)--cluster.ctl" = cluster{"error":errorcluster}
  T53 = typedef "Scripting Server.lvlib/get_object_help (Reply Payload)--cluster.ctl" = cluster{"help_string":string, "error":errorcluster}
  T54 = typedef "Scripting Server.lvlib/get_allowed_paths (Reply Payload)--cluster.ctl" = cluster{"Allowed Paths":string, "error":errorcluster}
  T55 = typedef "Scripting Server.lvlib/Cleanup VI (Reply Payload)--cluster.ctl" = cluster{"result":string, "error":errorcluster}
  T56 = typedef "Scripting Server.lvlib/get_loop_conditional_terminal (Reply Payload)--cluster.ctl" = cluster{"conditional_terminal_id":i32, "error":errorcluster}
  T57 = typedef "Scripting Server.lvlib/show_conditional_terminal (Reply Payload)--cluster.ctl" = cluster{"error":errorcluster}
  T58 = typedef "Scripting Server.lvlib/get_loop_iteration_terminal (Reply Payload)--cluster.ctl" = cluster{"iteration_terminal_id":i32, "error":errorcluster}
  T59 = typedef "Scripting Server.lvlib/create_project (Reply Payload)--cluster.ctl" = cluster{"project_id":i32, "error":errorcluster}
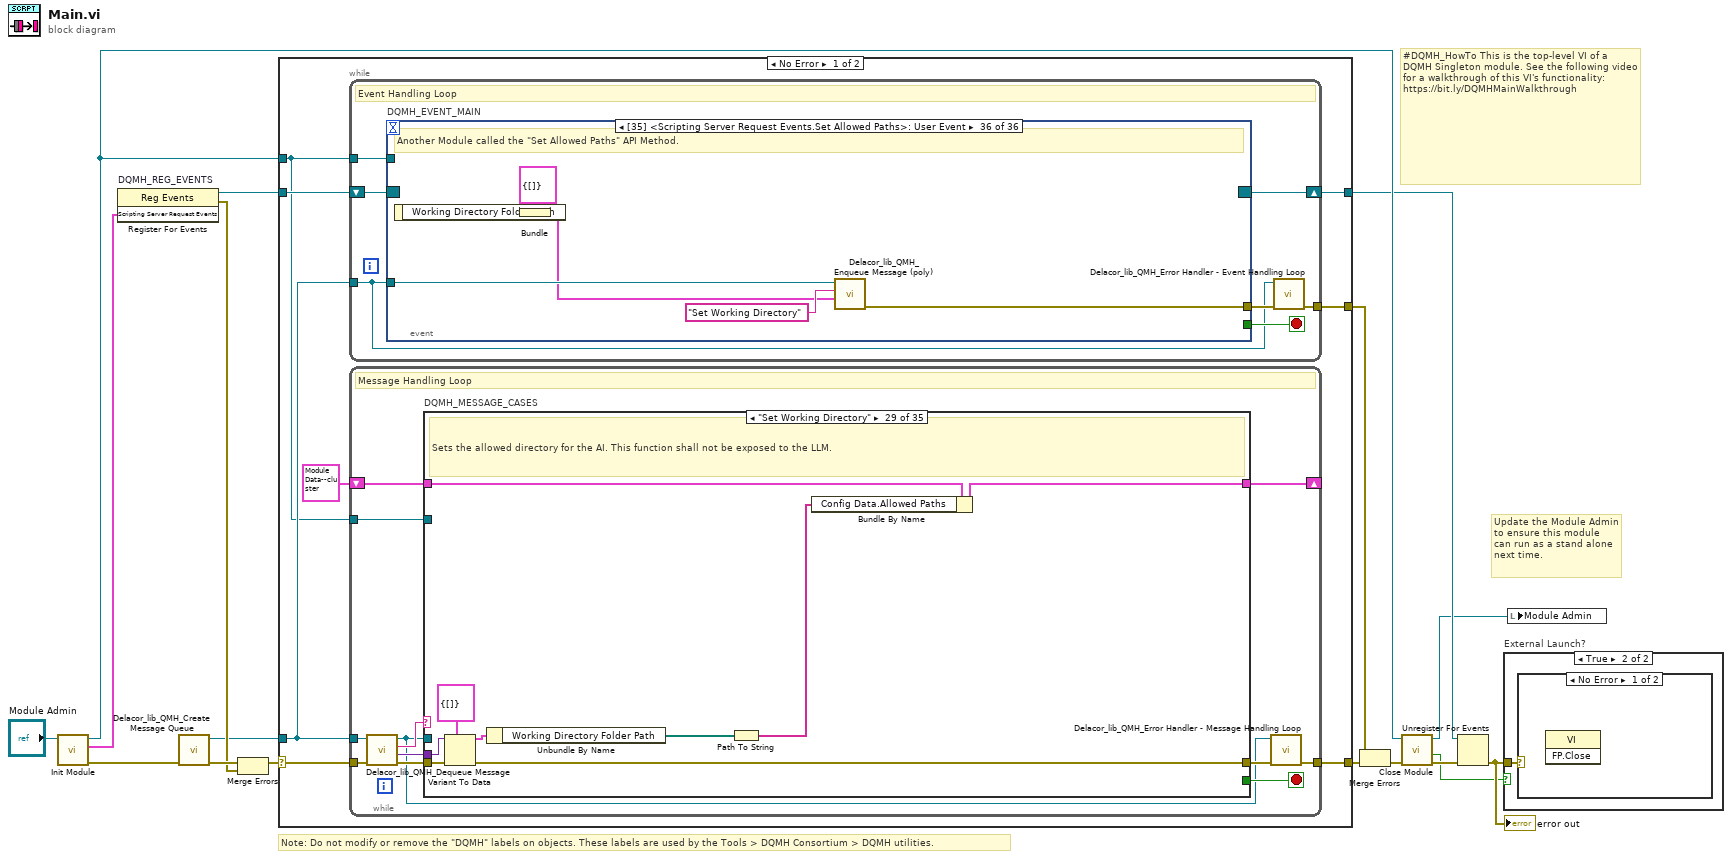
[diagram p0: block diagram]
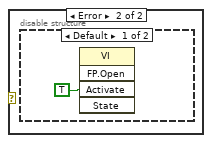
[diagram p3: hidden frame]
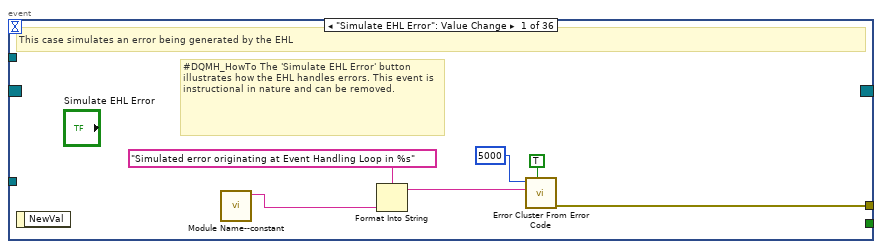
[diagram p5: hidden frame]
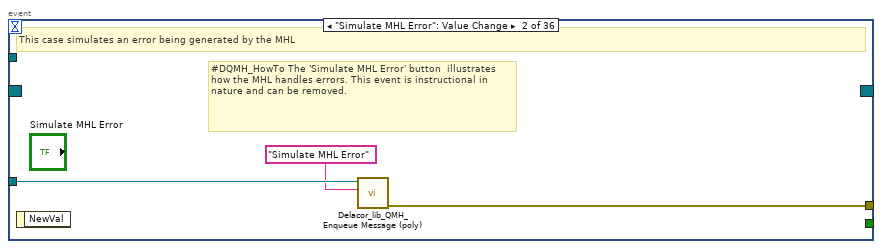
[diagram p6: hidden frame]
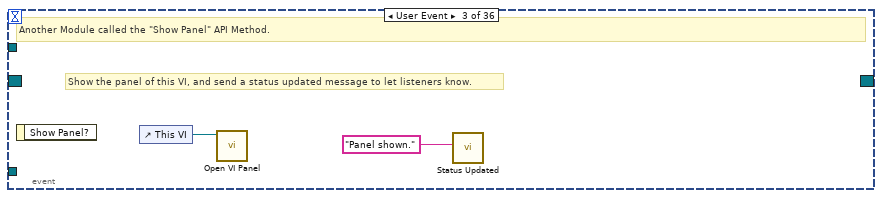
[diagram p7: hidden frame]
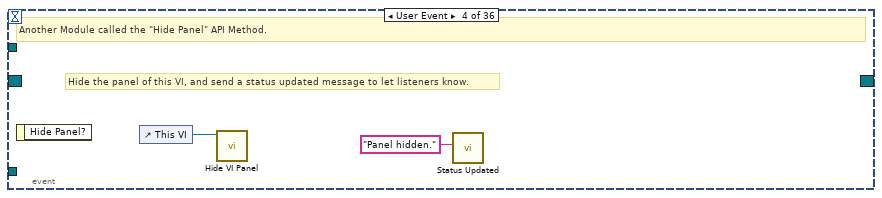
[diagram p8: hidden frame]
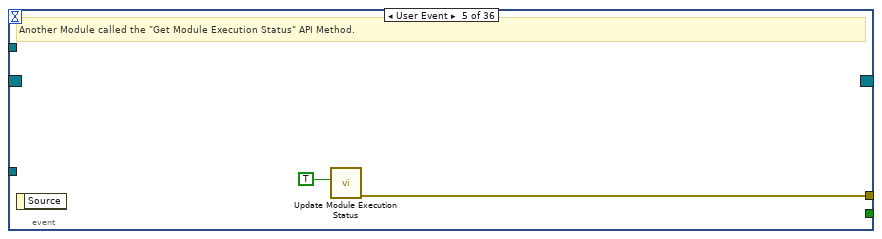
[diagram p9: hidden frame]
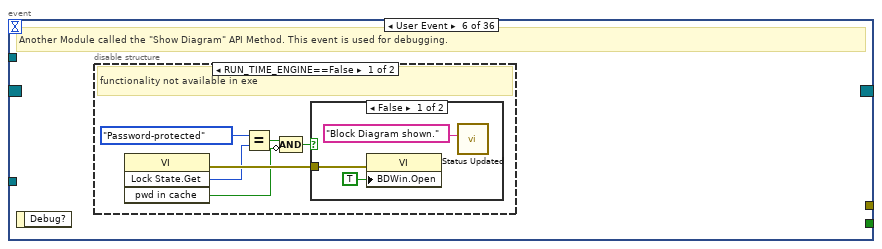
[diagram p10: hidden frame]
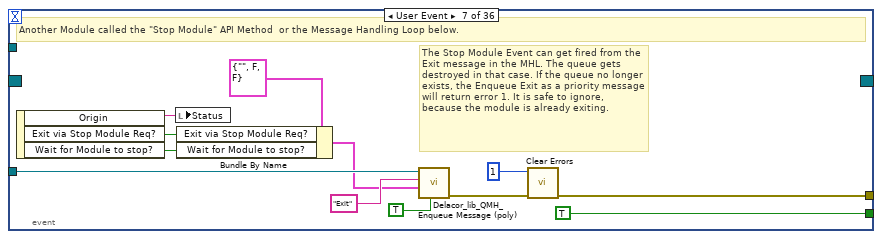
[diagram p13: hidden frame]
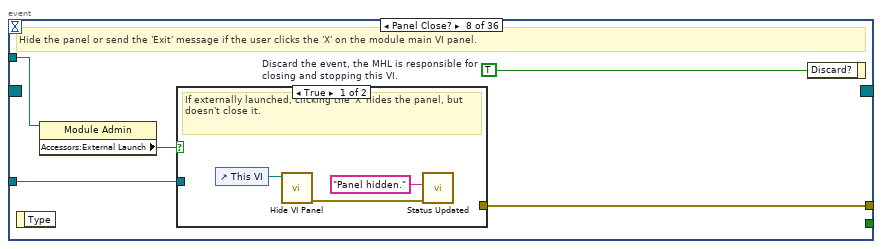
[diagram p14: hidden frame]
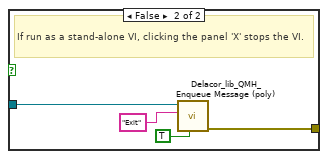
[diagram p15: hidden frame]
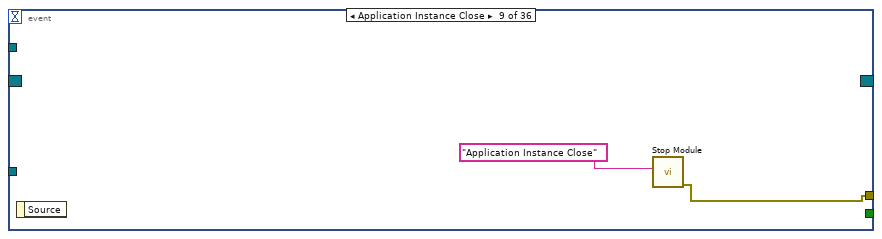
[diagram p16: hidden frame]
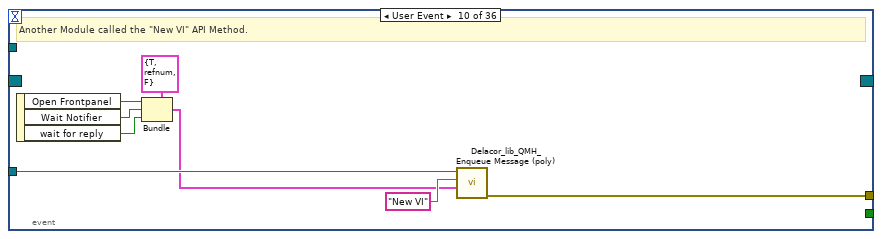
[diagram p17: hidden frame]
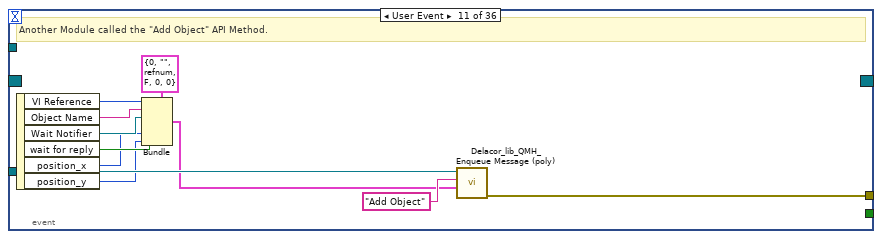
[diagram p18: hidden frame]
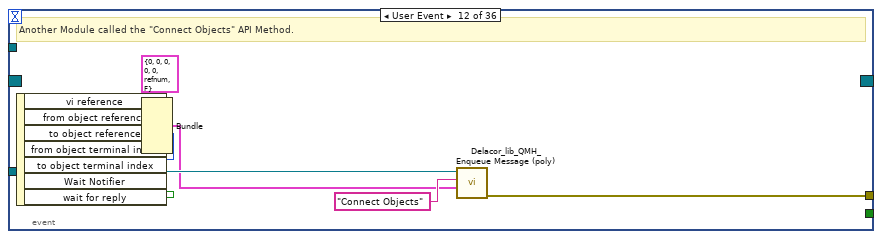
[diagram p19: hidden frame]
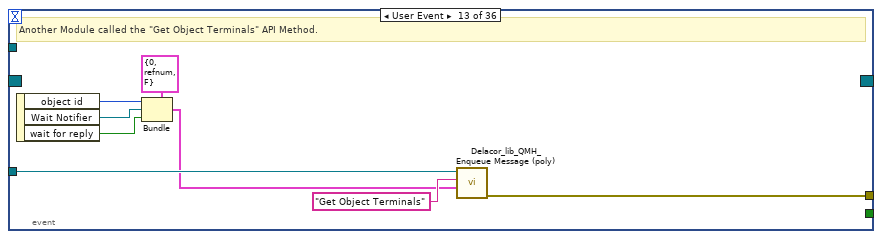
[diagram p20: hidden frame]
diagram:
  # "#DQMH_HowTo This is the top-level VI of a DQMH Singleton module. See the following video for a walkthrough of this VI's functionality: https://bit.ly/DQMHMainWalkthrough"
  # "Note: Do not modify or remove the \"DQMH\" labels on objects. These labels are used by the Tools > DQMH Consortium > DQMH utilities."
  # "Update the Module Admin to ensure this module can run as a stand alone next time."
  n1 = call "Init Module.vi"("Singleton Module Admin in"="Module Admin") -> ("error out"=w16:errorcluster, "Scripting Server Request Events"=w5:T1, "Singleton Module Admin out"=w8:refnum<class "Delacor_lib_QMH_Module Admin.lvclass">)  [unwired: 8 in]
  n2 = register-events "DQMH_REG_EVENTS"(w5) -> (reference out=w6:refnum<event-registration>, error out=w9:errorcluster)  [unwired: 2 in]
  n3 = call <vilib>:"Delacor_lib_QMH_Create Message Queue.vi"("error in"=w16) -> ("error out"=w11:errorcluster, "Message Queue"=w4:refnum<class "Delacor_lib_QMH_Message Queue.lvclass">)  [unwired: 9 in]
  n4 = Merge Errors(w11, w9) -> (w10:errorcluster)
  n5 = case shown="No Error" w10 {
    selector: w10 -> [w23 w796]
    tunnel: [w25 w795] -> w17
    tunnel: [w22 w794] -> w7
    tunnel: w6 -> [w20 w794]
    tunnel: w4 -> [w19 w789]
    tunnel: [w24 _] -> w14
    tunnel: w8 -> [w18 w790]
    frame No Error {
      n6 = while {
        tunnel: w19 -> [w26]
        shift-right: [w29] -> w22
        shift-left: w20 -> [w30]
        tunnel: [w31] -> w24
        tunnel: w18 -> [w27]
        stop <- w28 stop-if-true
        # "Event Handling Loop"
        n7 = event "DQMH_EVENT_MAIN" shown="[35] <Scripting Server Request Events.Set Allowed Paths>: User Event" {
          selector: w30 -> [_ _ _ _ _ _ _ _ _ _ _ _ _ _ _ _ _ _ _ _ _ _ _ _ _ _ _ _ _ _ _ _ _ _ _ _]
          dyn-events: [_ _ _ _ _ _ _ _ _ _ _ _ _ _ _ _ _ _ _ _ _ _ _ _ _ _ _ _ _ _ _ _ _ _ _ _] -> w29
          timeout: _ -> [_ _ _ _ _ _ _ _ _ _ _ _ _ _ _ _ _ _ _ _ _ _ _ _ _ _ _ _ _ _ _ _ _ _ _ _]
          tunnel: [_ _ _ _ _ _ TRUE ("Discard?") _ _ _ _ _ _ _ _ _ _ _ _ _ _ _ _ _ _ _ _ _ _ _ _ _ _ _ _ _] -> w28
          tunnel: w26 -> [_ w40 _ _ _ _ w64 w71 _ w90 w101 w113 w121 w129 w137 w147 w156 w165 w173 w182 w191 w201 w210 w218 w227 w236 w245 w254 w262 w270 w279 w287 w293 w300 w308 w314]
          tunnel: [w38 w41 _ _ w47 _ w67 w73 w82 w83 w95 w102 w114 w122 w130 w138 w148 w158 w167 w174 w183 w193 w202 w211 w219 w228 w237 w246 w255 w263 w271 w280 w288 w294 w301 w309] -> w32
          tunnel: w27 -> [_ _ _ _ _ _ _ w70 _ _ _ _ _ _ _ _ _ _ _ _ _ _ _ _ _ _ _ _ _ _ _ _ _ _ _ _]
          event "Simulate EHL Error": Value Change {
            # "#DQMH_HowTo The 'Simulate EHL Error' button  illustrates how the EHL handles errors. This event is instructional in nature and can be removed."
            # "This case simulates an error being generated by the EHL"
            n8 = event-data() -> ()  [unwired: 1 in, 1 out]
            n9 = call "Module Name--constant.vi"() -> ("Module Name"=w35:string)  [unwired: 11 in]
            n10 = Format Into String(format string="Simulated error originating at Event Handling Loop in %s", w35) -> (resulting string=w36:string)  [unwired: 2 in, 1 out]
            n11 = call <vilib>:"Error Cluster From Error Code.vi"("show call chain? (False)"=TRUE, "error message (\"\")"=w36, "error code (0)"=5000) -> ("error out"=w38:errorcluster)  [unwired: 6 in]
          }
          event "Simulate MHL Error": Value Change {
            # "#DQMH_HowTo The 'Simulate MHL Error' button  illustrates how the MHL handles errors. This event is instructional in nature and can be removed."
            # "This case simulates an error being generated by the MHL"
            n12 = event-data() -> ()  [unwired: 1 in, 1 out]
            n13 = call-poly <vilib>:"Delacor_lib_QMH_Enqueue Message (poly).vi"("Message"="Simulate MHL Error", "Message Queue in"=w40) -> ("error out"=w41:errorcluster)  [unwired: 8 in, 1 out]
          }
          event User Event {
            # "Show the panel of this VI, and send a status updated message to let listeners know."
            # "Another Module called the \"Show Panel\" API Method."
            n14 = event-data() -> ()  [unwired: 1 in, 1 out]
            n15 = control-ref of="This VI"() -> (w43:refnum<vi>)
            n16 = call "Open VI Panel.vi"("VI"=w43) -> ()  [unwired: 10 in, 1 out]
            n17 = call "Status Updated.vi"("Status"="Panel shown." ("format string")) -> ()  [unwired: 10 in, 1 out]
          }
          event User Event {
            # "Hide the panel of this VI, and send a status updated message to let listeners know."
            # "Another Module called the \"Hide Panel\" API Method."
            n18 = event-data() -> ()  [unwired: 1 in, 1 out]
            n19 = control-ref of="This VI"() -> (w45:refnum<vi>)
            n20 = call "Hide VI Panel.vi"("VI"=w45) -> ()  [unwired: 10 in, 1 out]
            n21 = call "Status Updated.vi"("Status"="Panel hidden." ("format string")) -> ()  [unwired: 10 in, 1 out]
          }
          event User Event {
            # "Another Module called the \"Get Module Execution Status\" API Method."
            n22 = event-data() -> ()  [unwired: 1 in, 1 out]
            n23 = call "Update Module Execution Status.vi"("Running?"=TRUE) -> ("error out"=w47:errorcluster)  [unwired: 10 in]
          }
          event User Event {
            # "Another Module called the \"Show Diagram\" API Method. This event is used for debugging."
            n24 = event-data() -> ()  [unwired: 1 in, 1 out]
            n25 = disable-structure shown="RUN_TIME_ENGINE==False" {
              frame condition #0 (active) {
                # "functionality not available in exe"
                n26 = invoke on="Invoke Node" class="VI" method="Lock State.Get"() -> (error out=w53:errorcluster, "Get Lock State"=w52:T4, "pwd in cache"=w49:bool)  [unwired: 4 in, 1 out]
                n27 = Equal?(x=T4."Password-protected", y=w52) -> (x = y?=w50:bool)
                n28 = Compound Arithmetic op=AND(w50, invert w49) -> (w48:bool)
                n29 = case shown="False" w48 {
                  tunnel: w53 -> [w56 _]
                  frame False {
                    n30 = property on="Property Node" class="VI"(error in=w56, "BDWin.Open"=TRUE ("Block Diagram Window:Open")) -> ()  [unwired: 1 in, 2 out]
                    n31 = call "Status Updated.vi"("Status"="Block Diagram shown." ("format string")) -> ()  [unwired: 10 in, 1 out]
                  }
                  frame True {
                    # "Password-protected VI, and the password is not in the cache. Do not show the diagram."
                  }
                }
              }
              frame condition #1 {
              }
            }
          }
          event User Event {
            # "The Stop Module Event can get fired from the Exit message in the MHL. The queue gets destroyed in that case. If the queue no longer exists, the Enqueue Exit as a priority message will return error 1. It is safe to ignore, because the module is already exiting."
            # "Another Module called the \"Stop Module\" API Method  or the Message Handling Loop below."
            n32 = event-data() -> ("Origin"=w63:string, "Exit via Stop Module Req?"=w59:bool, "Wait for Module to stop?"=w58:bool)  [unwired: 1 in]
            n33 = local write "Status"(w63) -> ()
            n34 = Bundle By Name(cluster=T5 {"Origin"="", "Exit via Stop Module Req?"=FALSE, "Wait for Module to stop?"=FALSE} ("Stop Argument"), "Exit via Stop Module Req?"=w59, "Wait for Module to stop?"=w58) -> (w57:T5)
            n35 = call-poly <vilib>:"Delacor_lib_QMH_Enqueue Message (poly).vi"("Priority Message? (F)"=TRUE, "Message Data"=w57, "Message"="Exit", "Message Queue in"=w64) -> ("error out"=w68:errorcluster)  [unwired: 6 in, 1 out]
            n36 = call <vilib>:"Clear Errors.vi"("error in (no error)"=w68, "specific error code to clear (0: all)"=1) -> ("error out"=w67:errorcluster)  [unwired: 4 in, 1 out]
          }
          event Panel Close? {
            w72 = TRUE  # Discard the event, the MHL is responsible for closing and stopping this VI.
            # "Hide the panel or send the 'Exit' message if the user clicks the 'X' on the module main VI panel."
            n37 = event-data() -> ()  [unwired: 1 in, 1 out]
            n38 = property on="Property Node" class="Module Admin"(reference=w70) -> ("Accessors:External Launch"=w69:bool)  [unwired: 1 in, 2 out]
            n39 = case shown="True" w69 {
              tunnel: w71 -> [_ w79]
              tunnel: [_ w80] -> w73
              frame True {
                # "If externally launched, clicking the 'X' hides the panel, but doesn't close it."
                n40 = control-ref of="This VI"() -> (w76:refnum<vi>)
                n41 = call "Hide VI Panel.vi"("VI"=w76) -> ("error out"=w74:errorcluster)  [unwired: 10 in]
                n42 = call "Status Updated.vi"("error in"=w74, "Status"="Panel hidden." ("format string")) -> ()  [unwired: 9 in, 1 out]
              }
              frame False {
                # "If run as a stand-alone VI, clicking the panel 'X' stops the VI."
                n43 = call-poly <vilib>:"Delacor_lib_QMH_Enqueue Message (poly).vi"("Priority Message? (F)"=TRUE, "Message"="Exit", "Message Queue in"=w79) -> ("error out"=w80:errorcluster)  [unwired: 7 in, 1 out]
              }
            }
            n44 = event-data ("Event Filter Node")("Discard?"=w72) -> ()  [unwired: 1 in, 1 out]
          }
          event Application Instance Close {
            n45 = event-data() -> ()  [unwired: 1 in, 1 out]
            n46 = call "Stop Module.vi"("Origin"="Application Instance Close") -> ("error out"=w82:errorcluster)  [unwired: 10 in]
          }
          event User Event {
            # "Another Module called the \"New VI\" API Method."
            n47 = event-data() -> ("Open Frontpanel"=w86:bool, "Wait Notifier"=w85:refnum<notifier>, "wait for reply"=w84:bool)  [unwired: 1 in]
            n48 = Bundle(cluster=T6 {"Open Frontpanel"=TRUE, "Wait Notifier"=refnum, "wait for reply"=FALSE} ("New VI Argument"), "Open Frontpanel"=w86, "Wait Notifier"=w85, "wait for reply"=w84) -> (w87:T6)
            n49 = call-poly <vilib>:"Delacor_lib_QMH_Enqueue Message (poly).vi"("Message Data"=w87, "Message"="New VI", "Message Queue in"=w90) -> ("error out"=w83:errorcluster)  [unwired: 7 in, 1 out]
          }
          event User Event {
            # "Another Module called the \"Add Object\" API Method."
            n50 = event-data() -> ("VI Reference"=w97:i32, "Object Name"=w96:string, "Wait Notifier"=w94:refnum<notifier>, "wait for reply"=w93:bool, "position_x"=w92:i32, "position_y"=w91:i32)  [unwired: 1 in]
            n51 = Bundle(cluster=T7 {"VI Reference"=0, "Object Name"="", "Wait Notifier"=refnum, "wait for reply"=FALSE, "position_x"=0, "position_y"=0} ("Add Object Argument"), "VI Reference"=w97, "Object Name"=w96, "Wait Notifier"=w94, "wait for reply"=w93, "position_x"=w92, "position_y"=w91) -> (w98:T7)
            n52 = call-poly <vilib>:"Delacor_lib_QMH_Enqueue Message (poly).vi"("Message Data"=w98, "Message"="Add Object", "Message Queue in"=w101) -> ("error out"=w95:errorcluster)  [unwired: 7 in, 1 out]
          }
          event User Event {
            # "Another Module called the \"Connect Objects\" API Method."
            n53 = event-data() -> ("vi reference"=w109:i32, "from object reference"=w108:i32, "to object reference"=w107:i32, "from object terminal index"=w106:i32, "to object terminal index"=w105:i32, "Wait Notifier"=w104:refnum<notifier>, "wait for reply"=w103:bool)  [unwired: 1 in]
            n54 = Bundle(cluster=T8 {"vi reference"=0, "from object reference"=0, "to object reference"=0, "from object terminal index"=0, "to object terminal index"=0, "Wait Notifier"=refnum, "wait for reply"=FALSE} ("Connect Objects Argument"), "vi reference"=w109, "from object reference"=w108, "to object reference"=w107, "from object terminal index"=w106, "to object terminal index"=w105, "Wait Notifier"=w104, "wait for reply"=w103) -> (w110:T8)
            n55 = call-poly <vilib>:"Delacor_lib_QMH_Enqueue Message (poly).vi"("Message Data"=w110, "Message"="Connect Objects", "Message Queue in"=w113) -> ("error out"=w102:errorcluster)  [unwired: 7 in, 1 out]
          }
          event User Event {
            # "Another Module called the \"Get Object Terminals\" API Method."
            n56 = event-data() -> ("object id"=w117:i32, "Wait Notifier"=w116:refnum<notifier>, "wait for reply"=w115:bool)  [unwired: 1 in]
            n57 = Bundle(cluster=T9 {"object id"=0, "Wait Notifier"=refnum, "wait for reply"=FALSE} ("Get Object Terminals Argument"), "object id"=w117, "Wait Notifier"=w116, "wait for reply"=w115) -> (w118:T9)
            n58 = call-poly <vilib>:"Delacor_lib_QMH_Enqueue Message (poly).vi"("Message Data"=w118, "Message"="Get Object Terminals", "Message Queue in"=w121) -> ("error out"=w114:errorcluster)  [unwired: 7 in, 1 out]
          }
          event User Event {
            # "Another Module called the \"get vi error list\" API Method."
            n59 = event-data() -> ("vi id"=w125:i32, "Wait Notifier"=w124:refnum<notifier>, "wait for reply"=w123:bool)  [unwired: 1 in]
            n60 = Bundle(cluster=T10 {"vi id"=0, "Wait Notifier"=refnum, "wait for reply"=FALSE} ("get vi error list Argument"), "vi id"=w125, "Wait Notifier"=w124, "wait for reply"=w123) -> (w126:T10)
            n61 = call-poly <vilib>:"Delacor_lib_QMH_Enqueue Message (poly).vi"("Message Data"=w126, "Message"="get vi error list", "Message Queue in"=w129) -> ("error out"=w122:errorcluster)  [unwired: 7 in, 1 out]
          }
          event User Event {
            # "Another Module called the \"Cleanup VI\" API Method."
            n62 = event-data() -> ("vi reference"=w133:i32, "Wait Notifier"=w132:refnum<notifier>, "wait for reply"=w131:bool)  [unwired: 1 in]
            n63 = Bundle(cluster=T11 {"vi reference"=0, "Wait Notifier"=refnum, "wait for reply"=FALSE} ("Cleanup VI Argument"), "vi reference"=w133, "Wait Notifier"=w132, "wait for reply"=w131) -> (w134:T11)
            n64 = call-poly <vilib>:"Delacor_lib_QMH_Enqueue Message (poly).vi"("Message Data"=w134, "Message"="Cleanup VI", "Message Queue in"=w137) -> ("error out"=w130:errorcluster)  [unwired: 7 in, 1 out]
          }
          event User Event {
            # "Another Module called the \"create_control\" API Method."
            n65 = event-data() -> ("Object ID"=w143:i32, "Terminal Index"=w142:i32, "Constant"=w141:bool, "Wait Notifier"=w140:refnum<notifier>, "wait for reply"=w139:bool)  [unwired: 1 in]
            n66 = Bundle(cluster=T12 {"Object ID"=0, "Terminal Index"=0, "Constant"=FALSE, "Wait Notifier"=refnum, "wait for reply"=FALSE, "Value"=""} ("create_control Argument"), "Object ID"=w143, "Terminal Index"=w142, "Constant"=w141, "Wait Notifier"=w140, "wait for reply"=w139) -> (w144:T12)  [unwired: 1 in]
            n67 = call-poly <vilib>:"Delacor_lib_QMH_Enqueue Message (poly).vi"("Message Data"=w144, "Message"="create_control", "Message Queue in"=w147) -> ("error out"=w138:errorcluster)  [unwired: 7 in, 1 out]
          }
          event User Event {
            # "Another Module called the \"Run VI\" API Method."
            n68 = event-data() -> ("VI ID"=w152:i32, "open_frontpanel"=w151:bool, "Wait Notifier"=w150:refnum<notifier>, "wait for reply"=w149:bool)  [unwired: 1 in]
            n69 = Bundle(cluster=T13 {"VI ID"=0, "open_frontpanel"=FALSE, "Wait Notifier"=refnum, "wait for reply"=FALSE} ("Run VI Argument"), "VI ID"=w152, "open_frontpanel"=w151, "Wait Notifier"=w150, "wait for reply"=w149) -> (w153:T13)
            n70 = call-poly <vilib>:"Delacor_lib_QMH_Enqueue Message (poly).vi"("Message Data"=w153, "Message"="Run VI", "Message Queue in"=w156) -> ("error out"=w148:errorcluster)  [unwired: 7 in, 1 out]
          }
          event User Event {
            # "Another Module called the \"add_to_selection\" API Method."
            n71 = event-data() -> ("object_id"=w161:i32, "Wait Notifier"=w160:refnum<notifier>, "wait for reply"=w159:bool, "vi_id"=w157:i32)  [unwired: 1 in]
            n72 = Bundle(cluster=T14 {"object_id"=0, "Wait Notifier"=refnum, "wait for reply"=FALSE, "vi_id"=0} ("add_to_selection Argument"), "object_id"=w161, "Wait Notifier"=w160, "wait for reply"=w159, "vi_id"=w157) -> (w162:T14)
            n73 = call-poly <vilib>:"Delacor_lib_QMH_Enqueue Message (poly).vi"("Message Data"=w162, "Message"="add_to_selection", "Message Queue in"=w165) -> ("error out"=w158:errorcluster)  [unwired: 7 in, 1 out]
          }
          event User Event {
            # "Another Module called the \"clear_selection_list\" API Method."
            n74 = event-data() -> ("Wait Notifier"=w169:refnum<notifier>, "wait for reply"=w168:bool, "vi_id"=w166:i32)  [unwired: 1 in]
            n75 = Bundle(cluster=T15 {"Wait Notifier"=refnum, "wait for reply"=FALSE, "vi_id"=0} ("clear_selection_list Argument"), "Wait Notifier"=w169, "wait for reply"=w168, "vi_id"=w166) -> (w170:T15)
            n76 = call-poly <vilib>:"Delacor_lib_QMH_Enqueue Message (poly).vi"("Message Data"=w170, "Message"="clear_selection_list", "Message Queue in"=w173) -> ("error out"=w167:errorcluster)  [unwired: 7 in, 1 out]
          }
          event User Event {
            # "Another Module called the \"remove_from_selection\" API Method."
            n77 = event-data() -> ("vi_id"=w178:i32, "object_id"=w177:i32, "Wait Notifier"=w176:refnum<notifier>, "wait for reply"=w175:bool)  [unwired: 1 in]
            n78 = Bundle(cluster=T16 {"vi_id"=0, "object_id"=0, "Wait Notifier"=refnum, "wait for reply"=FALSE} ("remove_from_selection Argument"), "vi_id"=w178, "object_id"=w177, "Wait Notifier"=w176, "wait for reply"=w175) -> (w179:T16)
            n79 = call-poly <vilib>:"Delacor_lib_QMH_Enqueue Message (poly).vi"("Message Data"=w179, "Message"="remove_from_selection", "Message Queue in"=w182) -> ("error out"=w174:errorcluster)  [unwired: 7 in, 1 out]
          }
          event User Event {
            # "Another Module called the \"enclose_selection\" API Method."
            n80 = event-data() -> ("vi_id"=w187:i32, "structure_type"=w186:string, "Wait Notifier"=w185:refnum<notifier>, "wait for reply"=w184:bool)  [unwired: 1 in]
            n81 = Bundle(cluster=T17 {"vi_id"=0, "structure_type"="", "Wait Notifier"=refnum, "wait for reply"=FALSE} ("enclose_selection Argument"), "vi_id"=w187, "structure_type"=w186, "Wait Notifier"=w185, "wait for reply"=w184) -> (w188:T17)
            n82 = call-poly <vilib>:"Delacor_lib_QMH_Enqueue Message (poly).vi"("Message Data"=w188, "Message"="enclose_selection", "Message Queue in"=w191) -> ("error out"=w183:errorcluster)  [unwired: 7 in, 1 out]
          }
          event User Event {
            # "Another Module called the \"rename_object\" API Method."
            n83 = event-data() -> ("new_label_name"=w197:string, "label_visible"=w196:bool, "Wait Notifier"=w195:refnum<notifier>, "wait for reply"=w194:bool, "object_id"=w192:i32)  [unwired: 1 in]
            n84 = Bundle(cluster=T18 {"new_label_name"="", "label_visible"=FALSE, "Wait Notifier"=refnum, "wait for reply"=FALSE, "object_id"=0} ("rename_object Argument"), "new_label_name"=w197, "label_visible"=w196, "Wait Notifier"=w195, "wait for reply"=w194, "object_id"=w192) -> (w198:T18)
            n85 = call-poly <vilib>:"Delacor_lib_QMH_Enqueue Message (poly).vi"("Message Data"=w198, "Message"="rename_object", "Message Queue in"=w201) -> ("error out"=w193:errorcluster)  [unwired: 7 in, 1 out]
          }
          event User Event {
            # "Another Module called the \"set_value\" API Method."
            n86 = event-data() -> ("object_id"=w206:i32, "value"=w205:string, "Wait Notifier"=w204:refnum<notifier>, "wait for reply"=w203:bool)  [unwired: 1 in]
            n87 = Bundle(cluster=T19 {"object_id"=0, "value"="", "Wait Notifier"=refnum, "wait for reply"=FALSE} ("set_value Argument"), "object_id"=w206, "value"=w205, "Wait Notifier"=w204, "wait for reply"=w203) -> (w207:T19)
            n88 = call-poly <vilib>:"Delacor_lib_QMH_Enqueue Message (poly).vi"("Message Data"=w207, "Message"="set_value", "Message Queue in"=w210) -> ("error out"=w202:errorcluster)  [unwired: 7 in, 1 out]
          }
          event User Event {
            # "Another Module called the \"delete_object\" API Method."
            n89 = event-data() -> ("object_id"=w214:i32, "Wait Notifier"=w213:refnum<notifier>, "wait for reply"=w212:bool)  [unwired: 1 in]
            n90 = Bundle(cluster=T20 {"object_id"=0, "Wait Notifier"=refnum, "wait for reply"=FALSE} ("delete_object Argument"), "object_id"=w214, "Wait Notifier"=w213, "wait for reply"=w212) -> (w215:T20)
            n91 = call-poly <vilib>:"Delacor_lib_QMH_Enqueue Message (poly).vi"("Message Data"=w215, "Message"="delete_object", "Message Queue in"=w218) -> ("error out"=w211:errorcluster)  [unwired: 7 in, 1 out]
          }
          event User Event {
            # "Another Module called the \"save_vi\" API Method."
            n92 = event-data() -> ("vi_id"=w223:i32, "path"=w222:string, "Wait Notifier"=w221:refnum<notifier>, "wait for reply"=w220:bool)  [unwired: 1 in]
            n93 = Bundle(cluster=T21 {"vi_id"=0, "path"="", "Wait Notifier"=refnum, "wait for reply"=FALSE} ("save_vi Argument"), "vi_id"=w223, "path"=w222, "Wait Notifier"=w221, "wait for reply"=w220) -> (w224:T21)
            n94 = call-poly <vilib>:"Delacor_lib_QMH_Enqueue Message (poly).vi"("Message Data"=w224, "Message"="save_vi", "Message Queue in"=w227) -> ("error out"=w219:errorcluster)  [unwired: 7 in, 1 out]
          }
          event User Event {
            # "Another Module called the \"get_structure_diagram\" API Method."
            n95 = event-data() -> ("structure_id"=w232:i32, "index"=w231:i32, "Wait Notifier"=w230:refnum<notifier>, "wait for reply"=w229:bool)  [unwired: 1 in]
            n96 = Bundle(cluster=T22 {"structure_id"=0, "index"=0, "Wait Notifier"=refnum, "wait for reply"=FALSE} ("get_structure_diagram Argument"), "structure_id"=w232, "index"=w231, "Wait Notifier"=w230, "wait for reply"=w229) -> (w233:T22)
            n97 = call-poly <vilib>:"Delacor_lib_QMH_Enqueue Message (poly).vi"("Message Data"=w233, "Message"="get_structure_diagram", "Message Queue in"=w236) -> ("error out"=w228:errorcluster)  [unwired: 7 in, 1 out]
          }
          event User Event {
            # "Another Module called the \"add_subvi\" API Method."
            n98 = event-data() -> ("diagram_id"=w241:i32, "subvi_path"=w240:string, "Wait Notifier"=w239:refnum<notifier>, "wait for reply"=w238:bool)  [unwired: 1 in]
            n99 = Bundle(cluster=T23 {"diagram_id"=0, "subvi_path"="", "Wait Notifier"=refnum, "wait for reply"=FALSE, "position_x"=0, "position_y"=0} ("add_subvi Argument"), "diagram_id"=w241, "subvi_path"=w240, "Wait Notifier"=w239, "wait for reply"=w238) -> (w242:T23)  [unwired: 2 in]
            n100 = call-poly <vilib>:"Delacor_lib_QMH_Enqueue Message (poly).vi"("Message Data"=w242, "Message"="add_subvi", "Message Queue in"=w245) -> ("error out"=w237:errorcluster)  [unwired: 7 in, 1 out]
          }
          event User Event {
            # "Another Module called the \"connect_to_pane\" API Method."
            n101 = event-data() -> ("control_id"=w250:i32, "connector_pane_index"=w249:i32, "Wait Notifier"=w248:refnum<notifier>, "wait for reply"=w247:bool)  [unwired: 1 in]
            n102 = Bundle(cluster=T24 {"control_id"=0, "connector_pane_index"=0, "Wait Notifier"=refnum, "wait for reply"=FALSE} ("connect_to_pane Argument"), "control_id"=w250, "connector_pane_index"=w249, "Wait Notifier"=w248, "wait for reply"=w247) -> (w251:T24)
            n103 = call-poly <vilib>:"Delacor_lib_QMH_Enqueue Message (poly).vi"("Message Data"=w251, "Message"="connect_to_pane", "Message Queue in"=w254) -> ("error out"=w246:errorcluster)  [unwired: 7 in, 1 out]
          }
          event User Event {
            # "Another Module called the \"get_object_help\" API Method."
            n104 = event-data() -> ("object_id"=w258:i32, "Wait Notifier"=w257:refnum<notifier>, "wait for reply"=w256:bool)  [unwired: 1 in]
            n105 = Bundle(cluster=T25 {"object_id"=0, "Wait Notifier"=refnum, "wait for reply"=FALSE} ("get_object_help Argument"), "object_id"=w258, "Wait Notifier"=w257, "wait for reply"=w256) -> (w259:T25)
            n106 = call-poly <vilib>:"Delacor_lib_QMH_Enqueue Message (poly).vi"("Message Data"=w259, "Message"="get_object_help", "Message Queue in"=w262) -> ("error out"=w255:errorcluster)  [unwired: 7 in, 1 out]
          }
          event User Event {
            # "Another Module called the \"get_loop_conditional_terminal\" API Method."
            n107 = event-data() -> ("loop_id"=w266:i32, "Wait Notifier"=w265:refnum<notifier>, "wait for reply"=w264:bool)  [unwired: 1 in]
            n108 = Bundle(cluster=T26 {"loop_id"=0, "Wait Notifier"=refnum, "wait for reply"=FALSE} ("get_loop_conditional_terminal Argument"), "loop_id"=w266, "Wait Notifier"=w265, "wait for reply"=w264) -> (w267:T26)
            n109 = call-poly <vilib>:"Delacor_lib_QMH_Enqueue Message (poly).vi"("Message Data"=w267, "Message"="get_loop_conditional_terminal", "Message Queue in"=w270) -> ("error out"=w263:errorcluster)  [unwired: 7 in, 1 out]
          }
          event User Event {
            # "Another Module called the \"show_conditional_terminal\" API Method."
            n110 = event-data() -> ("loop_id"=w275:i32, "show"=w274:bool, "Wait Notifier"=w273:refnum<notifier>, "wait for reply"=w272:bool)  [unwired: 1 in]
            n111 = Bundle(cluster=T27 {"loop_id"=0, "show"=FALSE, "Wait Notifier"=refnum, "wait for reply"=FALSE} ("show_conditional_terminal Argument"), "loop_id"=w275, "show"=w274, "Wait Notifier"=w273, "wait for reply"=w272) -> (w276:T27)
            n112 = call-poly <vilib>:"Delacor_lib_QMH_Enqueue Message (poly).vi"("Message Data"=w276, "Message"="show_conditional_terminal", "Message Queue in"=w279) -> ("error out"=w271:errorcluster)  [unwired: 7 in, 1 out]
          }
          event User Event {
            # "Another Module called the \"get_loop_iteration_terminal\" API Method."
            n113 = event-data() -> ("loop_id"=w283:i32, "Wait Notifier"=w282:refnum<notifier>, "wait for reply"=w281:bool)  [unwired: 1 in]
            n114 = Bundle(cluster=T28 {"loop_id"=0, "Wait Notifier"=refnum, "wait for reply"=FALSE} ("get_loop_iteration_terminal Argument"), "loop_id"=w283, "Wait Notifier"=w282, "wait for reply"=w281) -> (w284:T28)
            n115 = call-poly <vilib>:"Delacor_lib_QMH_Enqueue Message (poly).vi"("Message Data"=w284, "Message"="get_loop_iteration_terminal", "Message Queue in"=w287) -> ("error out"=w280:errorcluster)  [unwired: 7 in, 1 out]
          }
          event User Event {
            # "Another Module called the \"Read Config Data\" API Method."
            n116 = event-data() -> ("Boolean"=w289:bool)  [unwired: 1 in]
            n117 = Bundle(cluster=T29 {"Boolean"=FALSE} ("Read Config Data Argument"), "Boolean"=w289) -> (w290:T29)
            n118 = call-poly <vilib>:"Delacor_lib_QMH_Enqueue Message (poly).vi"("Message Data"=w290, "Message"="Read Config Data", "Message Queue in"=w293) -> ("error out"=w288:errorcluster)  [unwired: 7 in, 1 out]
          }
          event User Event {
            # "Another Module called the \"get_allowed_paths\" API Method."
            n119 = event-data() -> ("Wait Notifier"=w296:refnum<notifier>, "wait for reply"=w295:bool)  [unwired: 1 in]
            n120 = Bundle(cluster=T30 {"Wait Notifier"=refnum, "wait for reply"=FALSE} ("get_allowed_paths Argument"), "Wait Notifier"=w296, "wait for reply"=w295) -> (w297:T30)
            n121 = call-poly <vilib>:"Delacor_lib_QMH_Enqueue Message (poly).vi"("Message Data"=w297, "Message"="get_allowed_paths", "Message Queue in"=w300) -> ("error out"=w294:errorcluster)  [unwired: 7 in, 1 out]
          }
          event User Event {
            # "Another Module called the \"create_project\" API Method."
            n122 = event-data() -> ("File Path"=w304:string, "Wait Notifier"=w303:refnum<notifier>, "wait for reply"=w302:bool)  [unwired: 1 in]
            n123 = Bundle(cluster=T31 {"File Path"="", "Wait Notifier"=refnum, "wait for reply"=FALSE} ("create_project Argument"), "File Path"=w304, "Wait Notifier"=w303, "wait for reply"=w302) -> (w305:T31)
            n124 = call-poly <vilib>:"Delacor_lib_QMH_Enqueue Message (poly).vi"("Message Data"=w305, "Message"="create_project", "Message Queue in"=w308) -> ("error out"=w301:errorcluster)  [unwired: 7 in, 1 out]
          }
          event User Event {
            # "Another Module called the \"Set Allowed Paths\" API Method."
            n125 = event-data() -> ("Working Directory Folder Path"=w310:path[])  [unwired: 1 in]
            n126 = Bundle(cluster=T32 {"Working Directory Folder Path"=[]} ("Set Working Directory Argument"), "Working Directory Folder Path"=w310) -> (w311:T32)
            n127 = call-poly <vilib>:"Delacor_lib_QMH_Enqueue Message (poly).vi"("Message Data"=w311, "Message"="Set Working Directory", "Message Queue in"=w314) -> ("error out"=w309:errorcluster)  [unwired: 7 in, 1 out]
          }
        }
        n128 = call-dynamic "Delacor_lib_QMH_Error Handler - Event Handling Loop.vi"("error in"=w32, "Message Queue in"=w26) -> ("dup error in"=w31:errorcluster)  [unwired: 8 in, 1 out]
      }
      n129 = while {
        tunnel: w19 -> [w315]
        shift-right: [w323] -> _
        shift-left: T2 {"Status"="", "Current ID"=0, "References"=variant, "Config Data"={"Allowed Paths"=[]}} ("Data Cluster") -> [w324]
        tunnel: w23 -> [w326]
        tunnel: [w318] -> w25
        tunnel: w18 -> [w319]
        stop <- w322 stop-if-true
        # "Message Handling Loop"
        n130 = call-dynamic "Delacor_lib_QMH_Dequeue Message.vi"("error in"=w326, "Message Queue in"=w315) -> ("error out"=w325:errorcluster, "Message Data"=w320:variant, "Message"=w321:string, "Message Queue out"=w316:refnum<class "Delacor_lib_QMH_Message Queue.lvclass">)  [unwired: 6 in]
        n131 = case "DQMH_MESSAGE_CASES" shown="\"Set Working Directory\"" w321 {
          selector: w321 -> [_ _ _ _ _ _ _ _ _ _ _ _ _ _ _ _ _ _ _ _ _ _ _ _ _ _ _ _ _ _ _ _ _ _ w784]
          tunnel: w316 -> [_ _ _ _ _ _ _ _ _ _ _ _ _ _ _ _ _ _ _ _ _ _ _ _ _ _ _ _ _ _ _ _ w750 w772 _]
          tunnel: w325 -> [w345 w349 w364 w381 w395 w410 w425 w437 w452 w466 w480 w494 w508 w523 w537 w551 w565 w581 w596 w611 w625 w640 w653 w666 w679 w693 w705 w721 w732 w735 w737 w746 w757 w778 w787]
          tunnel: [w343 w349 w355 w369 w384 w398 w413 w428 w440 w455 w469 w483 w497 w513 w526 w540 w554 w570 w584 w599 w614 w629 w645 w658 w671 w687 w694 w713 w730 w734 w737 w745 w753 w773 w788] -> w317
          tunnel: w324 -> [w334 w348 w353 w370 w385 w409 w424 w436 w451 w465 w479 w493 w507 w522 w536 w550 w564 w580 w595 w610 w624 w639 w652 w665 w678 w685 w697 w720 w731 w733 w736 w743 w752 w771 w785]
          tunnel: [w333 w348 w354 w374 w388 w401 w416 w430 w444 w457 w472 w486 w499 w512 w529 w542 w557 w571 w588 w603 w617 w632 w643 w656 w669 w683 w697 w712 w726 w733 w736 w743 w752 w771 w785] -> w323
          tunnel: [_ _ _ _ _ _ _ _ _ _ _ _ _ _ _ _ _ _ _ _ _ _ _ _ _ _ _ _ _ _ _ _ _ w770 _] -> w322
          tunnel: w320 -> [_ _ w362 w380 w394 w408 w423 w435 w450 w464 w478 w492 w506 w521 w535 w549 w563 w578 w594 w609 w623 w638 w650 w663 w676 _ w704 w718 w729 _ _ _ w751 w769 _]
          tunnel: w319 -> [w335 _ _ _ _ _ _ _ _ _ _ _ _ _ _ _ _ _ _ _ _ _ _ _ _ _ _ _ _ _ _ _ w749 w764 _]
          frame "Initialize" {
            w329 = "Initial Message" ("Initial Message")
            # "Initialize - Any operation that needs to be done before the module can receive messages. Synchronize Caller Events.vi will inform Start Module.vi that the module has launched and is ready to receive messages. Module Did Init.vi will broadcast that the module initialized."
            n132 = call "Synchronize Caller Events.vi"("error in"=w345, "Singleton Module Admin in"=w335) -> ("error out"=w344:errorcluster, "Singleton Module Admin out"=w330:refnum<class "Delacor_lib_QMH_Module Admin.lvclass">)  [unwired: 8 in]
            n133 = property on="Property Node" class="Module Admin"(reference=w330) -> ("Accessors:External Launch"=w339:bool)  [unwired: 1 in, 2 out]
            n134 = Select(t=T34."Hidden" ("State"), s=w339, f=T34."Standard" ("State")) -> (s? t:f=w336:T34)
            n135 = call "Module Name--constant.vi"() -> ("Module Name"=w342:string)  [unwired: 11 in]
            n136 = property on="Property Node" class="VI"("Front Panel.Title"=w342) -> (reference out=w341:refnum<vi>, error out=w347:errorcluster)  [unwired: 2 in]
            n137 = invoke on="Invoke Node" class="VI" method="FP.Open"(reference=w341, error in=w347, "State"=w336) -> (reference out=w340:refnum<vi>, error out=w346:errorcluster)  [unwired: 2 in, 3 out]
            n138 = Bundle By Name(cluster=w334, "Status"=w329) -> (w333:T2)
            n139 = invoke on="Invoke Node" class="VI" method="FP.Center"(reference=w340, error in=w346) -> ()  [unwired: 1 in, 3 out]
            n140 = property on="Pane" class="Pane"("Origin"=T33 {"Horizontal"=0, "Vertical"=0}) -> ()  [unwired: 2 in, 2 out]
            n141 = call "Read Config Data.vi"("error in"=w344) -> ("error out"=w327:errorcluster)  [unwired: 10 in]
            n142 = call "Module Name--constant.vi"() -> ("Module Name"=w331:string)  [unwired: 11 in]
            n143 = call "Module Did Init.vi"("error in"=w327, "Initialized?"=TRUE, "Origin"=w331) -> ("error out"=w343:errorcluster)  [unwired: 8 in]
            "Status" <- w329
          }
          frame "---Module Specific---" {
            # "Separator -- The following cases handle messages specific to this Module."
          }
          frame "New VI" {
            # "Creates a new VI in the LabVIEW IDE. The VI Reference is stored and returned. This Reference can later be used to e.g. add modifications to the VI."
            n144 = Variant To Data(error in=w364, type=T6 {"Open Frontpanel"=TRUE, "Wait Notifier"=refnum, "wait for reply"=FALSE} ("New VI Argument"), Variant=w362) -> (data=w360:T6, error out=w363:errorcluster)
            n145 = Unbundle By Name(w360) -> ("Open Frontpanel"=w351:bool, "Wait Notifier"=w359:refnum<notifier>, "wait for reply"=w358:bool)
            n146 = call "Create New VI.vi"("Open Frontpanel"=w351, "Data Cluster in"=w353) -> ("message"=w352:string, "ID"=w350:i32, "Data Cluster out"=w354:T2)  [unwired: 7 in]
            n147 = Bundle By Name(cluster=T35 {"VI Reference"=0, "Result"="", "error"={"status"=FALSE, "code"=0, "source"=""}} ("New VI (Reply Payload)"), "Result"=w352, "VI Reference"=w350) -> (w357:T35)
            n148 = Merge Errors(w363) -> (w355:errorcluster)
            n149 = case "DQMH_FIRE_NOTIFIER" shown="True" w358 {
              tunnel: w359 -> [_ w366]
              tunnel: w357 -> [_ w365]
              frame False {
              }
              frame True {
                n150 = Send Notification(notification=w365, notifier=w366) -> ()  [unwired: 1 in, 2 out]
              }
            }
          }
          frame "Add Object" {
            # "Adds an object to the block diagram or frontpanel of the referenced vi. Get a VI reference from \"New VI\".\nAllowed object names are:\n.NET Container\n.NET Refnum\n2D Picture\n3D Picture\nAbsolute Value\nAccept TLS\nAccess Rights\nActiveX Container\nAdd\nAdd (with error terminals)\nAdd Array Elements\nAdd Entropy\nAdd Private Key To TLS Configuration\nAdd Trusted Certificate To TLS Configuration\nAgitator\nAllSpoll\nAlways Copy\nAnd\nAnd Array Elements\nAppend True/False String\nApplication Refnum\nArray (block diagram constant)\nArray (classic)\nArray (modern)\nArray Interface Control\nArray Max & Min\nArray of Strings to Path\nArray Size\nArray Subset\nArray To Cluster\nArray To Spreadsheet String\nArrayMemInfo\nAssert Structural Type Match\nAssert Structural Type Mismatch\nAtmospheric Tank (classic)\nAtmospheric Tank (modern)\nAutomation Close\nAutomation Open\nAutomation Refnum\nAvogadro Constant (1/mol)\nBase 10 Logarithm Of e\nBin #1\nBin #2\nBitpack to Array\nBluetooth Close Connection\nBluetooth Create Listener\nBluetooth Discover\nBluetooth Network Connection Refnum\nBluetooth Open Connection\nBluetooth Read\nBluetooth Wait On Listener\nBluetooth Write\nBoolean Array To Number\nBoolean To (0,1)\nBuild Array\nBuild Cluster Array\nBuild Map\nBuild Matrix\nBuild Path\nBuild Set\nBuild Waveform\nBundle\nBundle By Name\nByte Array To String\nByte Array To UTF-8 String\nByte Stream File Refnum\nCall By Reference\nCall Chain\nCall Library Function Node\nCall MATLAB Function\nCall Parent Class Method\nCAN Channel (block diagram constant)\nCAN Channel (classic)\nCAN Channel (modern)\nCAN Channel (system)\nCAN Interface (block diagram constant)\nCAN Interface (classic)\nCAN Interface (modern)\nCAN Interface (system)\nCAN Task (block diagram constant)\nCAN Task (classic)\nCAN Task (modern)\nCAN Task (system)\nCancel Button (modern)\nCancel Button (system)\nCancel Notification\nCarriage Return Constant\nCase Structure\nCast Unit Bases\nCheck Valve\nCheckbox (classic)\nCheckBox (modern)\nCheckbox (system)\nClass Specifier Constant\nClassic Color Box\nClassic Color Ramp\nClassic Horizontal Slide Switch\nClassic Vertical Slide\nClear Fixed-Point Overflow Status\nClose File\nClose File (deprecated)\nClose MATLAB Session\nClose Python Session\nClose Reference\nClose TLS Configuration\nClose Variable Connection\nClosure Structure\nCluster (classic)\nCluster (modern)\nCluster Constant\nCluster To Array\nCode Interface Node\nCoerce To Type\nCollection Size\nColor Box Constant\nColor Box Thin Border\nColored Rectangle (broken?)\nCombo Box (classic)\nCombo Box (modern)\nCombo Box (system)\nCombo Box Constant\nComplex Conjugate\nComplex To Polar\nComplex To Re/Im\nCompound Arithmetic\nCompressor\nConcatenate Strings\nConditional Disable Structure\nConstructor Node\nControl & Simulation Loop\nControl Help Window\nControl Online Help\nControl Refnum\nConvert Unit\nConveyer\nCopy\nCopy (deprecated)\nCosecant\nCosine\nCotangent\nCPU Information\nCreate Folder\nCreate Network Stream Endpoint\nCreate Network Stream Reader Endpoint\nCreate Network Stream Writer Endpoint\nCreate Stream\nCreate Unique Network Stream Endpoint\nCreate Unique Network Stream Reader Endpoint\nCreate Unique Network Stream Writer Endpoint\nCreate User Event\nCurrent Processor ID\nCurrent VI's Menubar\nCurrent VI's Path\nDAQmx Analog Trigger Source (block diagram constant)\nDAQmx Analog Trigger Source (classic)\nDAQmx Analog Trigger Source (modern)\nDAQmx Analog Trigger Source (system)\nDAQmx Device Name (block diagram constant)\nDAQmx Device Name (classic)\nDAQmx Device Name (modern)\nDAQmx Device Name (system)\nDAQmx Global Channel (block diagram constant)\nDAQmx Global Channel (classic)\nDAQmx Global Channel (modern)\nDAQmx Global Channel (system)\nDAQmx Physical Channel (block diagram constant)\nDAQmx Physical Channel (classic)\nDAQmx Physical Channel (modern)\nDAQmx Physical Channel (system)\nDAQmx Scale Name (block diagram constant)\nDAQmx Scale Name (classic)\nDAQmx Scale Name (modern)\nDAQmx Scale Name (system)\nDAQmx Switch (block diagram constant)\nDAQmx Switch (classic)\nDAQmx Switch (modern)\nDAQmx Switch (system)\nDAQmx Task Name (block diagram constant)\nDAQmx Task Name (classic)\nDAQmx Task Name (modern)\nDAQmx Task Name (system)\nDAQmx Terminal (block diagram constant)\nDAQmx Terminal (classic)\nDAQmx Terminal (modern)\nDAQmx Terminal (system)\nData Cache Size\nData Log File Refnum\nData Value Reference\nData Value Reference Constant\nDataSocket Close\nDataSocket Open\nDataSocket Read\nDataSocket Refnum\nDataSocket Write\nDate/Time To Seconds\nDecimal Digit?\nDecimal String To Number\nDecimate 1D Array\nDecomposeLockDataValRef\nDecomposeVariant\nDecrement\nDefault Directory\nDelete\nDelete (deprecated)\nDelete Data Value Reference\nDelete From Array\nDelete Menu Items\nDelete Variant Attribute\nDelete Waveform Attribute\nDeny Access\nDequeue Element\nDestroy Stream Endpoint\nDestroy User Event\nDevClear\nDevClearList\nDevice Control/Status\nDevice Refnum\nDiagram Disable Structure\nDial (classic)\nDial (modern)\nDigital Data (classic)\nDigital Data (modern)\nDigital Waveform Graph (classic)\nDigital Waveform Graph (modern)\nDirect Variable Read\nDirect Variable Write\nDivide\nDivide (with error terminals)\nDlg Horiz Scrollbar\nDlg Mac Group Box\nDlg Numeric #1\nDlg Numeric #2\nDlg String\nDlg Vert Scrollbar\nDown Arrow\nDown Bow Valve (flat)\nDown Bow Valve (outline)\nDown Bow Valve (shaded)\nDown Rect Valve (flat)\nDown Rect Valve (outline)\nDown Rect Valve (shaded)\nDown Tee (flat)\nDown Tee (shaded)\nDynamic FPGA Interface Cast\nEased Corner Rectangle\nElement of Set?\nElementary Charge (C)\nEmpty Array?\nEmpty Collection?\nEmpty Path Constant\nEmpty String Constant\nEmpty String/Path?\nEnable Menu Tracking\nEnableLocal\nEnableRemote\nEnd of Line Constant\nEnqueue Element\nEnqueue Element At Opposite End\nEnum (classic)\nEnum (modern)\nEnum (system)\nEnum Constant\nEOF\nEqual To 0?\nEqual?\nError Ring Constant\nEvent Callback Refnum\nEvent Data Node\nEvent Structure\nExchanger\nExclusive Or\nExponential\nExponential (Arg) -1\nExpression Node\nFalse Constant\nFeedback Node\nFieldPoint IO Point (block diagram constant)\nFieldPoint IO Point (classic)\nFieldPoint IO Point (modern)\nFIFO Refnum\nFile Dialog\nFile Dialog (deprecated)\nFile Path Control (classic)\nFile Path Control (modern)\nFile Path Control (system)\nFile Path Indicator (classic)\nFile Path Indicator (modern)\nFile/Directory Info\nFile/Directory Info (deprecated)\nFindLstn\nFindRQS\nFirst Call?\nFixed-Point Overflow?\nFixed-Point to Integer Cast\nFlat Box\nFlat Circle\nFlat Down Triangle\nFlat Frame\nFlat Left Triangle\nFlat Right Triangle\nFlat Round Button\nFlat Rounded Box\nFlat Sequence Structure\nFlat Square Button\nFlat Up Triangle\nFlatten To JSON\nFlatten To String\nFlatten To XML\nFlattened String To Variant\nFloating Point Equal?\nFlush Event Queue\nFlush File\nFlush File (deprecated)\nFlush Queue\nFlush Stream\nFor Loop\nFork\nFormat Date/Time String\nFormat Into File\nFormat Into String\nFormat Value\nFormula Node\nFPGA Refnum to Session\nFract/Exp String To Number\nFramed Color Box (classic)\nFramed Color Box (modern)\nFree Label\nFurnace\nGauge (classic)\nGauge (modern)\nGauge for Simon\nGenerate Front Panel Activity\nGenerate Occurrence\nGenerate User Event\nGenerate User-Defined Trace Event\nGet Control Values by Index\nGet Datalog Position\nGet Date/Time In Seconds\nGet Date/Time String\nGet Drag Drop Data\nGet File Position\nGet File Size\nGet Fixed-Point Components\nGet Help Window Status\nGet Matrix Diagonal\nGet Matrix Elements\nGet Menu Item Info\nGet Menu Selection\nGet Menu Short Cut Info\nGet Notifier Status\nGet Number of Records\nGet Permissions\nGet Queue Status\nGet Submatrix\nGet Type and Creator\nGet Variant Attribute\nGet Volume Info\nGet Waveform Attribute\nGet Waveform Components\nGlobal Variable\nGPIB Clear\nGPIB Initialization\nGPIB Misc\nGPIB Read\nGPIB Serial Poll\nGPIB Status\nGPIB Trigger\nGPIB Wait\nGPIB Write\nGravitational Constant (N m2/kg2)\nGreater Or Equal To 0?\nGreater Or Equal?\nGreater Than 0?\nGreater?\nHandle Peek\nHandle Poke\nHex Digit?\nHexadecimal String To Number\nHopper #1\nHopper #2\nHoriz Line\nHoriz Pipe (flat)\nHoriz Pipe (shaded)\nHorizontal Button Box\nHorizontal Fill Slide (classic)\nHorizontal Fill Slide (modern)\nHorizontal Gradient Oval\nHorizontal Gradient Rectangle\nHorizontal Gradient Rounded Rectangle\nHorizontal Graduated Bar\nHorizontal Pointer Slide (classic)\nHorizontal Pointer Slide (modern)\nHorizontal Pointer Slide (system)\nHorizontal Progress Bar (modern)\nHorizontal Progress Bar (system)\nHorizontal Scrollbar\nHorizontal Slide (classic)\nHorizontal Slide (system)\nHorizontal Smooth Box\nHorizontal Splitter Bar\nHorizontal Splitter Bar (Classic)\nHorizontal Splitter Bar (NXG Style)\nHorizontal Splitter Bar (System)\nHorizontal Switch\nHorizontal Tank\nHorizontal Toggle Switch (classic)\nHorizontal Toggle Switch (modern)\nHyperbolic Cosecant\nHyperbolic Cosine\nHyperbolic Cotangent\nHyperbolic Secant\nHyperbolic Sine\nHyperbolic Tangent\nIMAQ Session\nImplies\nIn Place Element Structure\nIn Range and Coerce\nInclude Fixed-Point Overflow Status\nIncrement\nIndex & Bundle Cluster Array\nIndex Array\nIndex String Array\nInitialize Array\nInline C Node\nInsert Into Array\nInsert Into Map\nInsert Into Set\nInsert Menu Items\nInteger to Fixed-Point Cast\nIntensity Chart (classic)\nIntensity Chart (modern)\nIntensity Graph (classic)\nIntensity Graph (modern)\nInterleave 1D Arrays\nInterpolate 1D Array\nInverse Cosecant\nInverse Cosine\nInverse Cotangent\nInverse Hyperbolic Cosecant\nInverse Hyperbolic Cosine\nInverse Hyperbolic Cotangent\nInverse Hyperbolic Secant\nInverse Hyperbolic Sine\nInverse Hyperbolic Tangent\nInverse Secant\nInverse Sine\nInverse Tangent\nInverse Tangent (2 Input)\nInvoke Node\nIP To String\nIrDA Close Connection\nIrDA Create Listener\nIrDA Discover\nIrDA Network Connection Refnum\nIrDA Open Connection\nIrDA Read\nIrDA Wait On Listener\nIrDA Write\nIsDebuggingActive\nIVI Delete Session\nIVI Logical Name (block diagram constant)\nIVI Logical Name (classic)\nIVI Logical Name (modern)\nIVI New Session\nJoin\nJoin Numbers\nJunction\nKnob (classic)\nKnob (modern)\nLabel (modern)\nLabel (system)\nLabeled Oblong Button\nLabeled Rectangular Button\nLabeled Round Button\nLabeled Square Button\nLabVIEW Object\nLeak Variant Value Reference\nLED Button\nLeft Arrow\nLeft Bow Valve (flat)\nLeft Bow Valve (outline)\nLeft Bow Valve (shaded)\nLeft Down Elbow (flat)\nLeft Down Elbow (shaded)\nLeft Pump (flat)\nLeft Pump (shaded)\nLeft Rect Valve (flat)\nLeft Rect Valve (outline)\nLeft Rect Valve (shaded)\nLeft Tee (flat)\nLeft Tee (shaded)\nLeft Up Elbow (flat)\nLeft Up Elbow (shaded)\nLess Or Equal To 0?\nLess Or Equal?\nLess Than 0?\nLess?\nLexical Class\nLine (chiseled, system)\nLine (chiseled, thick)\nLine (chiseled, thin)\nLine (thick)\nLine (thin)\nLine Feed Constant\nLine with Arrow (thick)\nLine with Arrow (thin)\nList Directory\nList Folder\nListbox (classic)\nListbox (modern)\nListbox (system)\nListbox Symbol Ring Constant\nLoad Certificates Into Memory\nLoad Private Key Into Memory\nLocal Variable\nLock Range\nLogarithm Base 10\nLogarithm Base 2\nLogarithm Base X\nLogical Shift\nLook In Map\nLookup Channel Probe\nLossy Enqueue Element\nLowered Box (thick)\nLowered Rounded Box\nMachine Epsilon\nMake TLS Configuration Immutable\nMakeAddr\nMantissa & Exponent\nMap\nMap Constant\nMatch First String\nMatch Pattern\nMatch True/False String\nMathScript Call By Reference\nMathScript Node\nMATLAB script\nMATLAB Session Refnum\nMatrix Size\nMax & Min\nMenu Refnum\nMenu Ring (classic)\nMenu Ring (modern)\nMenu-Popup Ring\nMerge Errors\nMerge Signals\nMeter (classic)\nMeter (modern)\nMixed Checkbox (system)\nMixed Signal Graph\nMolar Gas Constant (J/(mol K))\nMotion Resource (block diagram constant)\nMotion Resource (classic)\nMotion Resource (modern)\nMotor (flat)\nMotor (shaded)\nMove\nMove (deprecated)\nMulti-Segment Pipe\nMulticolumn Listbox (classic)\nMulticolumn Listbox (modern)\nMulticolumn Listbox (system)\nMultiply\nMultiply (with error terminals)\nMultiply Array Elements\nMultirate Structure\nNatural Logarithm\nNatural Logarithm (Arg +1)\nNatural Logarithm Base\nNatural Logarithm Of 10\nNatural Logarithm Of 2\nNatural Logarithm Of Pi\nNegate\nNegative Infinity\nNew Data Value Reference\nNew Directory\nNew File\nNew TLS Configuration\nNew VI\nNew VI Object\nNot\nNot A Number/Path/Refnum?\nNot A Path Constant\nNot a Refnum Constant\nNot a Shared Variable\nNot And\nNot Equal To 0?\nNot Equal?\nNot Exclusive Or\nNot Or\nNotifier Refnum\nNumber of Cache Levels\nNumber To Boolean Array\nNumber To Decimal String\nNumber To Engineering String\nNumber To Exponential String\nNumber To Fractional String\nNumber To Hexadecimal String\nNumber To Octal String\nNumeric Constant\nNumeric Control (classic)\nNumeric Control (modern)\nNumeric Control (system)\nNumeric Indicator (classic)\nNumeric Indicator (modern)\nObtain Notifier\nObtain Queue\nOccurrence Refnum\nOctal Digit?\nOctal String To Number\nOK Button (modern)\nOK Button (system)\nOld VISA Open\nOLE Variant\nOne Button Dialog\nOpen and Verify Variable Connection\nOpen Application Reference\nOpen Device\nOpen Dynamic Bitfile Reference\nOpen File\nOpen MATLAB Session\nOpen Python Session\nOpen Tank (flat classic)\nOpen Tank (shaded classic)\nOpen Variable Connection\nOpen Variable Connection in Background\nOpen VI Object Reference\nOpen VI Reference\nOpen/Create/Replace Datalog\nOpen/Create/Replace File\nOr\nOr Array Elements\nOval with Shadow\nPackage Matrix\nPassControl\nPath Constant\nPath to Array of Strings\nPath To String\nPath Type\nPi\nPi Divided By 2\nPi Multiplied By 2\nPick Line\nPict Ring (classic)\nPict Ring (modern)\nPict Ring (system)\nPixMap\nPixMap (warning: dangerous)\nPlanck's Constant (J/Hz)\nPlatform Flat Square Button\nPlug-In Control\nPolar To Complex\nPolar To Re/Im\nPositive Infinity\nPower Of 10\nPower Of 2\nPower Of X\nPPoll\nPPollConfig\nPPollUnconfig\nPreallocated Read from Binary File\nPreserve Run-Time Class\nPressure Tank (flat)\nPressure Tank (shaded)\nPreview Queue Element\nPrintable?\nProperty Node\nPulldown Menu Ring\nPush Button\nPython Node\nPython Session Refnum\nQueue Refnum\nQuit LabVIEW\nQuotient & Remainder\nRace Structure\nRadio Button (system)\nRadio Buttons (classic)\nRadio Buttons (modern)\nRadio Buttons (system)\nRaised Box (classic)\nRaised Box (modern)\nRaised Circle\nRaised Down Triangle\nRaised Frame\nRaised Left Triangle\nRaised Right Triangle\nRaised Rounded Box\nRaised Up Triangle\nRandom Number (0-1)\nRcvRespMsg\nRe-accept TLS\nRe/Im To Complex\nRe/Im To Polar\nRead Datalog\nRead Device\nRead File\nRead from Binary File\nRead from Text File\nRead Map Max & Min Keys\nRead Multiple Elements from Stream\nRead Set Max & Min\nRead Single Element from Stream\nRead Variable\nRead Variable with Timeout\nReadStatus\nReceive\nReceiveSetup\nRecessed Box\nRecessed Circle\nRecessed Down Triangle\nRecessed Frame (modern)\nRecessed Frame (system)\nRecessed Left Triangle\nRecessed Menu Ring\nRecessed Right Triangle\nRecessed Rounded Box\nRecessed Up Triangle\nReciprocal\nReciprocal Of e\nReciprocal Of Pi\nRecomposeUnlockDataValRef (warning: dangerous)\nRecomposeVariant (warning: dangerous)\nRectangular Stop Button\nRefnum to Path\nRefnum to Session\nRegion\nRegister Event Callback\nRegister For Events\nRegister Session\nRelease Notifier\nRelease Queue\nRemove Fixed-Point Overflow Status\nRemove From Map\nRemove From Set\nReplace Array Subset\nReplace Substring\nRequest Deallocation\nResetSys\nReshape Array\nResize Matrix\nResource Index\nReverse 1D Array\nReverse String\nRight Arrow\nRight Bow Valve (flat)\nRight Bow Valve (outline)\nRight Bow Valve (shaded)\nRight Down Elbow (flat)\nRight Down Elbow (shaded)\nRight Pump (flat)\nRight Pump (shaded)\nRight Rect Valve (flat)\nRight Rect Valve (outline)\nRight Rect Valve (shaded)\nRight Tee (flat)\nRight Tee (shaded)\nRight Up Elbow (flat)\nRight Up Elbow (shaded)\nRocker\nRotary Feeder\nRotate\nRotate 1D Array\nRotate Left With Carry\nRotate Right With Carry\nRotate String\nRound Button\nRound LED (classic)\nRound LED (modern)\nRound Light\nRound Push Button\nRound Push Button (profile)\nRound Radio Button\nRound Stop Button\nRound To Nearest\nRound Toward +Infinity\nRound Toward -Infinity\nRounded Rectangle with Shadow\nRT FIFO Create\nRT FIFO Delete\nRT FIFO Read\nRT FIFO Write\nRydberg Constant (1/m)\nScale By Power Of 2\nScan From File\nScan From String\nScan String For Tokens\nScan Value\nScanned Variable Read\nScanned Variable Write\nSearch 1D Array\nSearch and Replace String\nSearch Variable Container\nSearch/Split String\nSecant\nSeconds To Date/Time\nSeek\nSelect\nSend\nSend Notification\nSendCmds\nSendDataBytes\nSendIFC\nSendList\nSendLLO\nSendSetup\nSession to Refnum\nSet\nSet Constant\nSet Control Values by Index\nSet Datalog Position\nSet File Position\nSet File Size\nSet Matrix Diagonal\nSet Matrix Elements\nSet Menu Item Info\nSet Number of Records\nSet Occurrence\nSet Permissions\nSet Submatrix\nSet Type and Creator\nSet Variant Attribute\nSet Waveform Attribute\nSetRWLS\nSetTimeOut\nShared Variable\nShared Variable Constant\nShared Variable Control (classic)\nShared Variable Control (modern)\nShared Variable to String\nSign\nSimple Horizontal Slide\nSimple Numeric\nSimple String\nSimple Vertical Slide\nSinc\nSine\nSine & Cosine\nSize Handle\nSlide Switch\nSmoothed Oval\nSmoothed Rounded Rectangle\nSort 1D Array\nSort Array of String\nSpeed Of Light In Vacuum (m/sec)\nSpin Control (system)\nSplit 1D Array\nSplit Button\nSplit Number\nSplit Signals\nSpreadsheet String To Array\nSquare\nSquare Button\nSquare LED (classic)\nSquare LED (modern)\nSquare Light\nSquare Push Button\nSquare Push Button (profile)\nSquare Radio Button\nSquare Root\nStacked Sequence Structure\nStart TLS\nState\nState Diagram\nStatic VI Reference\nStop\nStop Button\nString Constant\nString Control (classic)\nString Control (modern)\nString Control (system)\nString Indicator (classic)\nString Indicator (modern)\nString Length\nString Subset\nString To Byte Array\nString To IP\nString To Path\nString to Shared Variable\nStrip Path\nSubPanel\nSubPanel (Classic)\nSubPanel (NXG Style)\nSubPanel (System)\nSubtract\nSubtract (with error terminals)\nSwap Bytes\nSwap Values\nSwap Vector Element\nSwap Words\nTab Constant\nTab Control (classic)\nTab Control (modern)\nTab Control (NXG Style)\nTab Control (system)\nTable (classic)\nTable (modern)\nTable (system)\nTag Attribute Ring\nTangent\nTank (classic)\nTank (modern)\nTarget Structure\nTCP Close Connection\nTCP Create Listener\nTCP Flattened Read\nTCP Flattened Write\nTCP Flex Read\nTCP Flex Write\nTCP Network Connection Refnum\nTCP Open Connection\nTCP Read\nTCP Wait On Listener\nTCP Write\nTDMS Advanced Asynchronous Read (Data Ref)\nTDMS Advanced Asynchronous Write (Data Ref)\nTDMS Close\nTDMS Configure Asynchronous Reads (Data Ref)\nTDMS Configure Asynchronous Writes (Data Ref)\nTDMS Defragment\nTDMS Delete Data\nTDMS File\nTDMS Flush\nTDMS Get Asynchronous Read Status (Data Ref)\nTDMS Get Asynchronous Write Status (Data Ref)\nTDMS Get Properties\nTDMS In Memory Close\nTDMS In Memory Open\nTDMS In Memory Read Bytes\nTDMS List Contents\nTDMS Open\nTDMS Read\nTDMS Refnum To File ID\nTDMS Set Properties\nTDMS Write\nTDMS Write IP\nTemporary Directory\nTestSRQ\nTestSys\nText & Pict Ring (classic)\nText & Pict Ring (modern)\nText Button\nText Ring (block diagram constant)\nText Ring (classic)\nText Ring (modern)\nText Ring (system)\nText to UTF-8\nThermometer (classic)\nThermometer (modern)\nThreshold 1D Array\nTick Count (ms)\nTime Stamp (block diagram constant)\nTime Stamp Control (classic)\nTime Stamp Control (modern)\nTime Stamp Control (system)\nTime Stamp Indicator (classic)\nTime Stamp Indicator (modern)\nTimed Loop\nTimed Sequence\nTLS configuration\nTLS Connection?\nTo Byte Integer\nTo Double Precision Complex\nTo Double Precision Float\nTo Extended Precision Complex\nTo Extended Precision Float\nTo Fixed-Point\nTo Long Integer\nTo Lower Case\nTo More Generic Class\nTo More Specific Class\nTo OLE Variant\nTo Probe String\nTo Quad Integer\nTo Single Precision Complex\nTo Single Precision Float\nTo Time Stamp\nTo Unsigned Byte Integer\nTo Unsigned Long Integer\nTo Unsigned Quad Integer\nTo Unsigned Word Integer\nTo Upper Case\nTo Variant\nTo Word Integer\nTraditional DAQ Channel (block diagram constant)\nTraditional DAQ Channel (classic)\nTraditional DAQ Channel (modern)\nTranspose 1D Array\nTranspose 2D Array\nTranspose Matrix\nTree (classic)\nTree (modern)\nTree (system)\nTrigger\nTriggerList\nTwo Button Dialog\nType and Creator\nType Cast\nType Error\nType Must Be Array\nType Must Be Cluster\nType Of\nType Specialization Structure\nUDP Close\nUDP Multicast Open\nUDP Network Connection Refnum\nUDP Open\nUDP Read\nUDP Write\nUnbitpack from Array\nUnbundle\nUnbundle By Name\nUnflatten From JSON\nUnflatten From String\nUnflatten From XML\nUnleak Variant Value Reference\nUnpackage Matrix\nUnregister For Events\nUnregister Session\nUp Arrow\nUp Bow Valve (flat)\nUp Bow Valve (outline)\nUp Bow Valve (shaded)\nUp Rect Valve (flat)\nUp Rect Valve (outline)\nUp Rect Valve (shaded)\nUp Tee (flat)\nUp Tee (shaded)\nUser Defined Refnum\nUser Defined Refnum Tag (block diagram constant)\nUser Defined Refnum Tag (classic)\nUser Defined Refnum Tag (modern)\nUser Defined Refnum Tag Flatten (classic)\nUser Defined Refnum Tag Flatten (modern)\nUser Defined Tag (block diagram constant)\nUser Defined Tag (classic)\nUser Defined Tag (modern)\nUser Item\nUTF-8 String To Byte Array\nUTF-8 to Text\nVariable Class Specifier Constant\nVariable Name Constant\nVariant\nVariant To Data\nVariant To Flattened String\nVert Line\nVert Pipe (flat)\nVert Pipe (shaded)\nVert Rocker\nVertical Fill Slide (classic)\nVertical Fill Slide (modern)\nVertical Gradient Oval\nVertical Gradient Rectangle\nVertical Gradient Rounded Rectangle\nVertical Graduated Bar\nVertical Pointer Slide (classic)\nVertical Pointer Slide (modern)\nVertical Pointer Slide (system)\nVertical Progress Bar (modern)\nVertical Progress Bar (system)\nVertical Scrollbar\nVertical Slide (system)\nVertical Slide Switch (classic)\nVertical Slide Switch (modern)\nVertical Smooth Box\nVertical Splitter Bar\nVertical Splitter Bar (Classic)\nVertical Splitter Bar (NXG Style)\nVertical Splitter Bar (System)\nVertical Switch\nVertical Toggle Switch (classic)\nVertical Toggle Switch (modern)\nVI Library\nVI Refnum\nVI Server Reference\nVISA Assert Interrupt Signal\nVISA Assert Trigger\nVISA Assert Utility Signal\nVISA Clear\nVISA Close\nVISA Disable Event\nVISA Discard Events\nVISA Enable Event\nVISA Find Resource\nVISA Flush I/O Buffer\nVISA GPIB Command\nVISA GPIB Control ATN\nVISA GPIB Control REN\nVISA GPIB Pass Control\nVISA GPIB Send IFC\nVISA In 16\nVISA In 32\nVISA In 64\nVISA In 8\nVISA Lock\nVISA Map Address\nVISA Map Trigger\nVISA Memory Allocation\nVISA Memory Allocation Ex\nVISA Memory Free\nVISA Move\nVISA Move In 16\nVISA Move In 32\nVISA Move In 64\nVISA Move In 8\nVISA Move Out 16\nVISA Move Out 32\nVISA Move Out 64\nVISA Move Out 8\nVISA Open\nVISA Out 16\nVISA Out 32\nVISA Out 64\nVISA Out 8\nVISA Peek 16\nVISA Peek 32\nVISA Peek 64\nVISA Peek 8\nVISA Poke 16\nVISA Poke 32\nVISA Poke 64\nVISA Poke 8\nVISA Read\nVISA Read STB\nVISA Read To File\nVISA Refnum to Session\nVISA Resource Name\nVISA resource name (classic)\nVISA resource name (modern)\nVISA Set I/O Buffer Size\nVISA Status Description\nVISA Unlock\nVISA Unmap Address\nVISA Unmap Trigger\nVISA USB Control In\nVISA USB Control Out\nVISA VXI Cmd or Query\nVISA Wait on Event\nVISA Write\nVISA Write From File\nVolume Info\nWait (ms)\nWait For Activity\nWait For Front Panel Activity\nWait for GPIB RQS\nWait on Notification\nWait on Notification from Multiple\nWait on Notification from Multiple with Notifier History\nWait on Notification with Notifier History\nWait on Occurrence\nWait Until Next ms Multiple\nWaitSRQ\nWaveform Chart\nWaveform Chart (classic)\nWaveform Chart (modern)\nWaveform Graph (classic)\nWaveform Graph (modern)\nWhile Loop #1\nWhile Loop #2\nWhite Space?\nWrite Datalog\nWrite Device\nWrite File\nWrite Multiple Elements to Stream\nWrite Single Element to Stream\nWrite to Binary File\nWrite to Text File\nWrite Variable\nWrite Variable with Timeout\nXY Graph (classic)\nXY Graph (modern)\nY-th Root of X"
            n151 = Variant To Data(error in=w381, type=T7 {"VI Reference"=0, "Object Name"="", "Wait Notifier"=refnum, "wait for reply"=FALSE, "position_x"=0, "position_y"=0} ("Add Object Argument"), Variant=w380) -> (data=w367:T7, error out=w369:errorcluster)
            n152 = Unbundle By Name(w367) -> ("Wait Notifier"=w378:refnum<notifier>, "wait for reply"=w377:bool)
            n153 = control-ref of="Ring 2"() -> (w371:refnum<vi>)
            n154 = call "add vi object.vi"("Ring in"=w371, "error in (no error)"=w369, "Add Object Argument"=w367, "Data Cluster in"=w370) -> ("error out"=w373:errorcluster, "Result"=w372:string, "object_id"=w368:i32, "Data Cluster out"=w374:T2)  [unwired: 4 in]
            n155 = Bundle By Name(cluster=T36 {"error"={"status"=FALSE, "code"=0, "source"=""}, "Object ID"=0, "Result"=""} ("Add Object (Reply Payload)"), "error"=w373, "Result"=w372, "Object ID"=w368) -> (w376:T36)
            n156 = case "DQMH_FIRE_NOTIFIER" shown="True" w377 {
              tunnel: w378 -> [_ w383]
              tunnel: w376 -> [_ w382]
              frame False {
              }
              frame True {
                n157 = Send Notification(notification=w382, notifier=w383) -> ()  [unwired: 1 in, 2 out]
              }
            }
          }
          frame "Connect Objects" {
            # "Connects two terminals of two objects with a wire on the block diagram of a labview vi. To get a new VI use \"new vi\" to add objects to a vi use \"add object\"."
            n158 = Variant To Data(error in=w395, type=T8 {"vi reference"=0, "from object reference"=0, "to object reference"=0, "from object terminal index"=0, "to object terminal index"=0, "Wait Notifier"=refnum, "wait for reply"=FALSE} ("Connect Objects Argument"), Variant=w394) -> (data=w386:T8, error out=w384:errorcluster)
            n159 = Unbundle By Name(w386) -> ("Wait Notifier"=w392:refnum<notifier>, "wait for reply"=w391:bool)
            n160 = call "Wire Two Objects.vi"("error in (no error)"=w384, "input cluster"=w386, "Data Cluster in"=w385) -> ("error out"=w387:errorcluster, "Data Cluster out"=w388:T2)  [unwired: 7 in]
            n161 = Bundle By Name(cluster=T37 {"result"="", "error"={"status"=FALSE, "code"=0, "source"=""}} ("Connect Objects (Reply Payload)"), "error"=w387) -> (w390:T37)
            n162 = case "DQMH_FIRE_NOTIFIER" shown="True" w391 {
              tunnel: w392 -> [_ w397]
              tunnel: w390 -> [_ w396]
              frame False {
              }
              frame True {
                n163 = Send Notification(notification=w396, notifier=w397) -> ()  [unwired: 1 in, 2 out]
              }
            }
          }
          frame "Get Object Terminals" {
            # "Returns the Terminals Names and/or descriptions as a string as well as their Index to be used in other functions like connect objects."
            n164 = Variant To Data(error in=w410, type=T9 {"object id"=0, "Wait Notifier"=refnum, "wait for reply"=FALSE} ("Get Object Terminals Argument"), Variant=w408) -> (data=w402:T9, error out=w398:errorcluster)
            n165 = Unbundle By Name(w402) -> ("Wait Notifier"=w406:refnum<notifier>, "wait for reply"=w405:bool)
            n166 = call "get terminal info.vi"("error in (no error)"=w398, "Get Object Terminals Argument"=w402, "Data Cluster in"=w409) -> ("error out"=w400:errorcluster, "String"=w399:string, "Data Cluster out"=w401:T2)  [unwired: 6 in]
            n167 = Bundle By Name(cluster=T38 {"terminals description"="", "error"={"status"=FALSE, "code"=0, "source"=""}} ("Get Object Terminals (Reply Payload)"), "terminals description"=w399, "error"=w400) -> (w404:T38)
            n168 = case "DQMH_FIRE_NOTIFIER" shown="True" w405 {
              tunnel: w406 -> [_ w412]
              tunnel: w404 -> [_ w411]
              frame False {
              }
              frame True {
                n169 = Send Notification(notification=w411, notifier=w412) -> ()  [unwired: 1 in, 2 out]
              }
            }
          }
          frame "get vi error list" {
            # "Returns the current error list (list you see when clicking the run arrow) in a text format giving information about what on the block diagram needs to be fixed. Use this to see if your actions worked."
            n170 = Variant To Data(error in=w425, type=T10 {"vi id"=0, "Wait Notifier"=refnum, "wait for reply"=FALSE} ("get vi error list Argument"), Variant=w423) -> (data=w417:T10, error out=w413:errorcluster)
            n171 = Unbundle By Name(w417) -> ("Wait Notifier"=w421:refnum<notifier>, "wait for reply"=w420:bool)  [unwired: 1 out]
            n172 = call "generate vi error list.vi"("error in (no error)"=w413, "get vi error list Argument"=w417, "Data Cluster in"=w424) -> ("error out"=w414:errorcluster, "Error Description"=w415:string, "Data Cluster out"=w416:T2)  [unwired: 6 in]
            n173 = Bundle By Name(cluster=T39 {"error list"="", "error"={"status"=FALSE, "code"=0, "source"=""}} ("get vi error list (Reply Payload)"), "error list"=w415, "error"=w414) -> (w419:T39)
            n174 = case "DQMH_FIRE_NOTIFIER" shown="True" w420 {
              tunnel: w421 -> [_ w427]
              tunnel: w419 -> [_ w426]
              frame False {
              }
              frame True {
                n175 = Send Notification(notification=w426, notifier=w427) -> ()  [unwired: 1 in, 2 out]
              }
            }
          }
          frame "Cleanup VI" {
            # "Cleans up the block diagram of a vi referenced by reference number."
            n176 = Variant To Data(error in=w437, type=T11 {"vi reference"=0, "Wait Notifier"=refnum, "wait for reply"=FALSE} ("Cleanup VI Argument"), Variant=w435) -> (data=w429:T11, error out=w428:errorcluster)
            n177 = Unbundle By Name(w429) -> ("Wait Notifier"=w433:refnum<notifier>, "wait for reply"=w432:bool)
            n178 = call "clean up vis blockdiagram.vi"("error in (no error)"=w428, "Cleanup VI Argument"=w429, "Data Cluster in"=w436) -> ("Cleanup VI (Reply Payload)"=w431:T55, "Data Cluster out"=w430:T2)  [unwired: 6 in, 1 out]
            n179 = case "DQMH_FIRE_NOTIFIER" shown="True" w432 {
              tunnel: w433 -> [_ w439]
              tunnel: w431 -> [_ w438]
              frame False {
              }
              frame True {
                n180 = Send Notification(notification=w438, notifier=w439) -> ()  [unwired: 1 in, 2 out]
              }
            }
          }
          frame "create_control" {
            # "Creates a control or indicator on the terminal specified by Object ID and Terminal Index, depending on if it's a in- or output of the node. If Constant is set to True, it can only be used on node inputs and will create a constant.\nIt will return the reference to the created control or indicator, that is a reference to the frontpanel element. If constant is True it returns a reference to the block diagram object (constant)."
            n181 = Variant To Data(error in=w452, type=T12 {"Object ID"=0, "Terminal Index"=0, "Constant"=FALSE, "Wait Notifier"=refnum, "wait for reply"=FALSE, "Value"=""} ("create_control Argument"), Variant=w450) -> (data=w443:T12, error out=w440:errorcluster)
            n182 = Unbundle By Name(w443) -> ("Wait Notifier"=w448:refnum<notifier>, "wait for reply"=w447:bool)  [unwired: 3 out]
            n183 = call "Do Create Control.vi"("error in (no error)"=w440, "create_control Argument"=w443, "Data Cluster in"=w451) -> ("error out"=w441:errorcluster, "new reference"=w442:i32, "Data Cluster out"=w444:T2)  [unwired: 6 in]
            n184 = Bundle By Name(cluster=T40 {"Object ID"=0, "error"={"status"=FALSE, "code"=0, "source"=""}} ("create_control (Reply Payload)"), "Object ID"=w442, "error"=w441) -> (w446:T40)
            n185 = case "DQMH_FIRE_NOTIFIER" shown="True" w447 {
              tunnel: w448 -> [_ w454]
              tunnel: w446 -> [_ w453]
              frame False {
              }
              frame True {
                n186 = Send Notification(notification=w453, notifier=w454) -> ()  [unwired: 1 in, 2 out]
              }
            }
          }
          frame "Run VI" {
            # "Runs a VI specified by VI ID and brings the frontpanel to foreground if open_frontpanel is set to True."
            n187 = Variant To Data(error in=w466, type=T13 {"VI ID"=0, "open_frontpanel"=FALSE, "Wait Notifier"=refnum, "wait for reply"=FALSE} ("Run VI Argument"), Variant=w464) -> (data=w458:T13, error out=w455:errorcluster)
            n188 = Unbundle By Name(w458) -> ("Wait Notifier"=w462:refnum<notifier>, "wait for reply"=w461:bool)
            n189 = call "Do Run VI.vi"("error in (no error)"=w455, "Run VI Argument"=w458, "Data Cluster in"=w465) -> ("error out"=w456:errorcluster, "Data Cluster out"=w457:T2)  [unwired: 7 in]
            n190 = Bundle By Name(cluster=T41 {"error"={"status"=FALSE, "code"=0, "source"=""}} ("Run VI (Reply Payload)"), "error"=w456) -> (w460:T41)
            n191 = case "DQMH_FIRE_NOTIFIER" shown="True" w461 {
              tunnel: w462 -> [_ w468]
              tunnel: w460 -> [_ w467]
              frame False {
              }
              frame True {
                n192 = Send Notification(notification=w467, notifier=w468) -> ()  [unwired: 1 in, 2 out]
              }
            }
          }
          frame "add_to_selection" {
            # "Adds an object specified by object_id to the selection list. Use this to copy & paste or enclose a selection. Use clear_selection or remove_from_selection to remove the object from the list. Make sure to check if the selection list looks good."
            n193 = Variant To Data(error in=w480, type=T14 {"object_id"=0, "Wait Notifier"=refnum, "wait for reply"=FALSE, "vi_id"=0} ("add_to_selection Argument"), Variant=w478) -> (data=w471:T14, error out=w469:errorcluster)
            n194 = Unbundle By Name(w471) -> ("Wait Notifier"=w476:refnum<notifier>, "wait for reply"=w475:bool)
            n195 = call "Do Add To Selection.vi"("error in (no error)"=w469, "add_to_selection Argument"=w471, "Data Cluster in"=w479) -> ("error out"=w470:errorcluster, "Data Cluster out"=w472:T2)  [unwired: 7 in]
            n196 = Bundle By Name(cluster=T42 {"Current Selection"=[], "error"={"status"=FALSE, "code"=0, "source"=""}} ("add_to_selection (Reply Payload)"), "error"=w470) -> (w474:T42)
            n197 = case "DQMH_FIRE_NOTIFIER" shown="True" w475 {
              tunnel: w476 -> [_ w482]
              tunnel: w474 -> [_ w481]
              frame False {
              }
              frame True {
                n198 = Send Notification(notification=w481, notifier=w482) -> ()  [unwired: 1 in, 2 out]
              }
            }
          }
          frame "clear_selection_list" {
            # "Clears all elements in the selection list. Use this before making a new selection."
            n199 = Variant To Data(error in=w494, type=T15 {"Wait Notifier"=refnum, "wait for reply"=FALSE, "vi_id"=0} ("clear_selection_list Argument"), Variant=w492) -> (data=w485:T15, error out=w483:errorcluster)
            n200 = Unbundle By Name(w485) -> ("Wait Notifier"=w490:refnum<notifier>, "wait for reply"=w489:bool)
            n201 = call "Do Clear Selection List.vi"("error in (no error)"=w483, "input cluster"=w485, "Data Cluster in"=w493) -> ("error out"=w484:errorcluster, "Data Cluster out"=w486:T2)  [unwired: 7 in]
            n202 = Bundle By Name(cluster=T43 {"error"={"status"=FALSE, "code"=0, "source"=""}} ("clear_selection_list (Reply Payload)"), "error"=w484) -> (w488:T43)
            n203 = case "DQMH_FIRE_NOTIFIER" shown="True" w489 {
              tunnel: w490 -> [_ w496]
              tunnel: w488 -> [_ w495]
              frame False {
              }
              frame True {
                n204 = Send Notification(notification=w495, notifier=w496) -> ()  [unwired: 1 in, 2 out]
              }
            }
          }
          frame "remove_from_selection" {
            # "Removes the object specified by object_id from the current selection list and returns the resulting new list."
            n205 = Variant To Data(error in=w508, type=T16 {"vi_id"=0, "object_id"=0, "Wait Notifier"=refnum, "wait for reply"=FALSE} ("remove_from_selection Argument"), Variant=w506) -> (data=w500:T16, error out=w497:errorcluster)
            n206 = Unbundle By Name(w500) -> ("Wait Notifier"=w504:refnum<notifier>, "wait for reply"=w503:bool)
            n207 = call "Do Remove From Selection.vi"("error in (no error)"=w497, "remove_from_selection Argument"=w500, "Data Cluster in"=w507) -> ("error out"=w498:errorcluster, "Data Cluster out"=w499:T2)  [unwired: 7 in]
            n208 = Bundle By Name(cluster=T44 {"current_selection"=[], "error"={"status"=FALSE, "code"=0, "source"=""}} ("remove_from_selection (Reply Payload)"), "error"=w498) -> (w502:T44)
            n209 = case "DQMH_FIRE_NOTIFIER" shown="True" w503 {
              tunnel: w504 -> [_ w510]
              tunnel: w502 -> [_ w509]
              frame False {
              }
              frame True {
                n210 = Send Notification(notification=w509, notifier=w510) -> ()  [unwired: 1 in, 2 out]
              }
            }
          }
          frame "enclose_selection" {
            # "Use this function to efficiently generate Loops or other structures around existing code. This is the quickest way to create loops including tunnles and wiring, wire the objects first, then create a loop around them, tunnles will be there automatically. Use the add_to_selection, remove_from_selection and clear_selection_list tools to change the current selection, connect_objects to connect them, then call this tool to create a structure around them.\nAllowed values for structure_type are:\nWhile Loop\nFor Loop\nCase Structure\nSequence Structure\nEvent Structure"
            n211 = Variant To Data(error in=w523, type=T17 {"vi_id"=0, "structure_type"="", "Wait Notifier"=refnum, "wait for reply"=FALSE} ("enclose_selection Argument"), Variant=w521) -> (data=w511:T17, error out=w513:errorcluster)
            n212 = Unbundle By Name(w511) -> ("Wait Notifier"=w519:refnum<notifier>, "wait for reply"=w518:bool)  [unwired: 2 out]
            n213 = call "Do Enclose Selection.vi"("error in (no error)"=w513, "enclose_selection Argument"=w511, "Data Cluster in"=w522) -> ("error out"=w514:errorcluster, "object_id"=w515:i32, "Data Cluster out"=w512:T2)  [unwired: 6 in]
            n214 = Bundle By Name(cluster=T45 {"object_id"=0, "error"={"status"=FALSE, "code"=0, "source"=""}} ("enclose_selection (Reply Payload)"), "object_id"=w515, "error"=w514) -> (w517:T45)
            n215 = case "DQMH_FIRE_NOTIFIER" shown="True" w518 {
              tunnel: w519 -> [_ w525]
              tunnel: w517 -> [_ w524]
              frame False {
              }
              frame True {
                n216 = Send Notification(notification=w524, notifier=w525) -> ()  [unwired: 1 in, 2 out]
              }
            }
          }
          frame "rename_object" {
            # "Use this to change an objects Label.Text property. Usually used for frontpanel objects. Use the label_visible True/False to decide if the label is displayed afterwards."
            n217 = Variant To Data(error in=w537, type=T18 {"new_label_name"="", "label_visible"=FALSE, "Wait Notifier"=refnum, "wait for reply"=FALSE, "object_id"=0} ("rename_object Argument"), Variant=w535) -> (data=w528:T18, error out=w526:errorcluster)
            n218 = Unbundle By Name(w528) -> ("Wait Notifier"=w533:refnum<notifier>, "wait for reply"=w532:bool)
            n219 = call "Do Rename Object.vi"("error in (no error)"=w526, "rename_object Argument"=w528, "Data Cluster in"=w536) -> ("error out"=w527:errorcluster, "Data Cluster out"=w529:T2)  [unwired: 7 in]
            n220 = Bundle By Name(cluster=T46 {"error"={"status"=FALSE, "code"=0, "source"=""}} ("rename_object (Reply Payload)"), "error"=w527) -> (w531:T46)
            n221 = case "DQMH_FIRE_NOTIFIER" shown="True" w532 {
              tunnel: w533 -> [_ w539]
              tunnel: w531 -> [_ w538]
              frame False {
              }
              frame True {
                n222 = Send Notification(notification=w538, notifier=w539) -> ()  [unwired: 1 in, 2 out]
              }
            }
          }
          frame "set_value" {
            # "Sets the value of a constant or control/indicator. The value is transferred as a string, but can be also a number."
            n223 = Variant To Data(error in=w551, type=T19 {"object_id"=0, "value"="", "Wait Notifier"=refnum, "wait for reply"=FALSE} ("set_value Argument"), Variant=w549) -> (data=w543:T19, error out=w540:errorcluster)
            n224 = Unbundle By Name(w543) -> ("Wait Notifier"=w547:refnum<notifier>, "wait for reply"=w546:bool)
            n225 = call "Do Set Value.vi"("error in (no error)"=w540, "set_value Argument"=w543, "Data Cluster in"=w550) -> ("error out"=w541:errorcluster, "Data Cluster out"=w542:T2)  [unwired: 7 in]
            n226 = Bundle By Name(cluster=T47 {"error"={"status"=FALSE, "code"=0, "source"=""}} ("set_value (Reply Payload)"), "error"=w541) -> (w545:T47)
            n227 = case "DQMH_FIRE_NOTIFIER" shown="True" w546 {
              tunnel: w547 -> [_ w553]
              tunnel: w545 -> [_ w552]
              frame False {
              }
              frame True {
                n228 = Send Notification(notification=w552, notifier=w553) -> ()  [unwired: 1 in, 2 out]
              }
            }
          }
          frame "delete_object" {
            # "removes the object from the blockdiagram or frontpanel."
            n229 = Variant To Data(error in=w565, type=T20 {"object_id"=0, "Wait Notifier"=refnum, "wait for reply"=FALSE} ("delete_object Argument"), Variant=w563) -> (data=w556:T20, error out=w554:errorcluster)
            n230 = Unbundle By Name(w556) -> ("Wait Notifier"=w561:refnum<notifier>, "wait for reply"=w560:bool)
            n231 = call "Do Delete Object.vi"("error in (no error)"=w554, "delete_object Argument"=w556, "Data Cluster in"=w564) -> ("error out"=w555:errorcluster, "Data Cluster out"=w557:T2)  [unwired: 7 in]
            n232 = Bundle By Name(cluster=T48 {"error"={"status"=FALSE, "code"=0, "source"=""}} ("delete_object (Reply Payload)"), "error"=w555) -> (w559:T48)
            n233 = case "DQMH_FIRE_NOTIFIER" shown="True" w560 {
              tunnel: w561 -> [_ w567]
              tunnel: w559 -> [_ w566]
              frame False {
              }
              frame True {
                n234 = Send Notification(notification=w566, notifier=w567) -> ()  [unwired: 1 in, 2 out]
              }
            }
          }
          frame "save_vi" {
            # "Saves a VI to the specified path. If Path is empty and vi was saved before, it saves to same location"
            n235 = Variant To Data(error in=w581, type=T21 {"vi_id"=0, "path"="", "Wait Notifier"=refnum, "wait for reply"=FALSE} ("save_vi Argument"), Variant=w578) -> (data=w572:T21, error out=w579:errorcluster)
            n236 = Unbundle By Name(w572) -> ("Wait Notifier"=w576:refnum<notifier>, "wait for reply"=w575:bool)
            n237 = call "Do Save VI.vi"("error in (no error)"=w579, "save_vi Argument"=w572, "Data Cluster in"=w580) -> ("error out"=w570:errorcluster, "VI Path"=w569:path, "Data Cluster out"=w571:T2)  [unwired: 6 in]
            n238 = Path To String(path=w569) -> (string=w568:string)
            n239 = Bundle By Name(cluster=T49 {"path_out"="", "error"={"status"=FALSE, "code"=0, "source"=""}} ("save_vi (Reply Payload)"), "path_out"=w568, "error"=w570) -> (w574:T49)
            n240 = case "DQMH_FIRE_NOTIFIER" shown="True" w575 {
              tunnel: w576 -> [_ w583]
              tunnel: w574 -> [_ w582]
              frame False {
              }
              frame True {
                n241 = Send Notification(notification=w582, notifier=w583) -> ()  [unwired: 1 in, 2 out]
              }
            }
          }
          frame "get_structure_diagram" {
            # "Returns the id of a sub-diagram of a structure (the inside of a loop or case-structure). Use this to add objects to a structure instead of to the top level blockdiagram. For Case-Structures, use the index option to iterate through them, for loops ignore index. Also consider using the \"enclose_selection\" tool if you work with structures to make wiring easier."
            n242 = Variant To Data(error in=w596, type=T22 {"structure_id"=0, "index"=0, "Wait Notifier"=refnum, "wait for reply"=FALSE} ("get_structure_diagram Argument"), Variant=w594) -> (data=w587:T22, error out=w584:errorcluster)
            n243 = Unbundle By Name(w587) -> ("Wait Notifier"=w592:refnum<notifier>, "wait for reply"=w591:bool)  [unwired: 2 out]
            n244 = call "Do Get Structure Diagram.vi"("error in (no error)"=w584, "get_structure_diagram Argument"=w587, "Data Cluster in"=w595) -> ("error out"=w585:errorcluster, "diagram_id"=w586:i32, "Data Cluster out"=w588:T2)  [unwired: 6 in]
            n245 = Bundle By Name(cluster=T50 {"diagram_id"=0, "error"={"status"=FALSE, "code"=0, "source"=""}} ("get_structure_diagram (Reply Payload)"), "diagram_id"=w586, "error"=w585) -> (w590:T50)
            n246 = case "DQMH_FIRE_NOTIFIER" shown="True" w591 {
              tunnel: w592 -> [_ w598]
              tunnel: w590 -> [_ w597]
              frame False {
              }
              frame True {
                n247 = Send Notification(notification=w597, notifier=w598) -> ()  [unwired: 1 in, 2 out]
              }
            }
          }
          frame "add_subvi" {
            # "Adds a SubVI to a blockdiagram or sturcture subdiagram similar to the add_object method."
            n248 = Variant To Data(error in=w611, type=T23 {"diagram_id"=0, "subvi_path"="", "Wait Notifier"=refnum, "wait for reply"=FALSE, "position_x"=0, "position_y"=0} ("add_subvi Argument"), Variant=w609) -> (data=w602:T23, error out=w599:errorcluster)
            n249 = Unbundle By Name(w602) -> ("Wait Notifier"=w607:refnum<notifier>, "wait for reply"=w606:bool)  [unwired: 2 out]
            n250 = call "Do Add Subvi.vi"("error in (no error)"=w599, "add_subvi Argument"=w602, "Data Cluster in"=w610) -> ("error out"=w600:errorcluster, "object_id"=w601:i32, "Data Cluster out"=w603:T2)  [unwired: 6 in]
            n251 = Bundle By Name(cluster=T51 {"subvi_id"=0, "error"={"status"=FALSE, "code"=0, "source"=""}} ("add_subvi (Reply Payload)"), "subvi_id"=w601, "error"=w600) -> (w605:T51)
            n252 = case "DQMH_FIRE_NOTIFIER" shown="True" w606 {
              tunnel: w607 -> [_ w613]
              tunnel: w605 -> [_ w612]
              frame False {
              }
              frame True {
                n253 = Send Notification(notification=w612, notifier=w613) -> ()  [unwired: 1 in, 2 out]
              }
            }
          }
          frame "connect_to_pane" {
            # "takes a control_id and connects the corresponding frontpanel control or indicator to the connector pane of the subvi. Do this to all necessary fronpanel controls/indicators to use the VI as a SubVI. The subvis by default have 4 fields on the left and right, and two on top/bottom. Their index starts at the bottom right, and goes counter clockwise."
            n254 = Variant To Data(error in=w625, type=T24 {"control_id"=0, "connector_pane_index"=0, "Wait Notifier"=refnum, "wait for reply"=FALSE} ("connect_to_pane Argument"), Variant=w623) -> (data=w616:T24, error out=w614:errorcluster)
            n255 = Unbundle By Name(w616) -> ("Wait Notifier"=w621:refnum<notifier>, "wait for reply"=w620:bool)  [unwired: 2 out]
            n256 = call "do connect to pane.vi"("error in (no error)"=w614, "connect_to_pane Argument"=w616, "Data Cluster in"=w624) -> ("error out"=w615:errorcluster, "Data Cluster out"=w617:T2)  [unwired: 7 in]
            n257 = Bundle By Name(cluster=T52 {"error"={"status"=FALSE, "code"=0, "source"=""}} ("connect_to_pane (Reply Payload)"), "error"=w615) -> (w619:T52)
            n258 = case "DQMH_FIRE_NOTIFIER" shown="True" w620 {
              tunnel: w621 -> [_ w627]
              tunnel: w619 -> [_ w626]
              frame False {
              }
              frame True {
                n259 = Send Notification(notification=w626, notifier=w627) -> ()  [unwired: 1 in, 2 out]
              }
            }
          }
          frame "get_object_help" {
            # "returns the labview detailed help article including termina descriptions. To get the exact indexes of the terminals use the get terminal info."
            n260 = Variant To Data(error in=w640, type=T25 {"object_id"=0, "Wait Notifier"=refnum, "wait for reply"=FALSE} ("get_object_help Argument"), Variant=w638) -> (data=w631:T25, error out=w629:errorcluster)
            n261 = Unbundle By Name(w631) -> ("Wait Notifier"=w636:refnum<notifier>, "wait for reply"=w635:bool)  [unwired: 1 out]
            n262 = call "Do Get Object Help.vi"("error in (no error)"=w629, "get_object_help Argument"=w631, "Data Cluster in"=w639) -> ("error out"=w628:errorcluster, "help_string"=w630:string, "Data Cluster out"=w632:T2)  [unwired: 6 in]
            n263 = Bundle By Name(cluster=T53 {"help_string"="", "error"={"status"=FALSE, "code"=0, "source"=""}} ("get_object_help (Reply Payload)"), "help_string"=w630, "error"=w628) -> (w634:T53)
            n264 = case "DQMH_FIRE_NOTIFIER" shown="True" w635 {
              tunnel: w636 -> [_ w642]
              tunnel: w634 -> [_ w641]
              frame False {
              }
              frame True {
                n265 = Send Notification(notification=w641, notifier=w642) -> ()  [unwired: 1 in, 2 out]
              }
            }
          }
          frame "get_loop_conditional_terminal" {
            # "Returns the conditional terminal of a while- or for-loop (if enabled), to be used with connect_objects (as to_object_id, with index 0)."
            n266 = Variant To Data(error in=w653, type=T26 {"loop_id"=0, "Wait Notifier"=refnum, "wait for reply"=FALSE} ("get_loop_conditional_terminal Argument"), Variant=w650) -> (data=w644:T26, error out=w651:errorcluster)
            n267 = Unbundle By Name(w644) -> ("Wait Notifier"=w648:refnum<notifier>, "wait for reply"=w647:bool)  [unwired: 1 out]
            n268 = call "Do Get Cond Terminal.vi"("error in (no error)"=w651, "get_loop_conditional_terminal Argument"=w644, "Data Cluster in"=w652) -> ("error out"=w645:errorcluster, "get_loop_conditional_terminal (Reply Payload)"=w646:T56, "Data Cluster out"=w643:T2)  [unwired: 6 in]
            n269 = case "DQMH_FIRE_NOTIFIER" shown="True" w647 {
              tunnel: w648 -> [_ w655]
              tunnel: w646 -> [_ w654]
              frame False {
              }
              frame True {
                n270 = Send Notification(notification=w654, notifier=w655) -> ()  [unwired: 1 in, 2 out]
              }
            }
          }
          frame "show_conditional_terminal" {
            # "Shows or hides the conditional terminal of a for loop."
            n271 = Variant To Data(error in=w666, type=T27 {"loop_id"=0, "show"=FALSE, "Wait Notifier"=refnum, "wait for reply"=FALSE} ("show_conditional_terminal Argument"), Variant=w663) -> (data=w657:T27, error out=w664:errorcluster)
            n272 = Unbundle By Name(w657) -> ("Wait Notifier"=w661:refnum<notifier>, "wait for reply"=w660:bool)  [unwired: 2 out]
            n273 = call "do show conditional terminal.vi"("error in (no error)"=w664, "show_conditional_terminal Argument"=w657, "Data Cluster in"=w665) -> ("error out"=w658:errorcluster, "show_conditional_terminal (Reply Payload)"=w659:T57, "Data Cluster out"=w656:T2)  [unwired: 6 in]
            n274 = case "DQMH_FIRE_NOTIFIER" shown="True" w660 {
              tunnel: w661 -> [_ w668]
              tunnel: w659 -> [_ w667]
              frame False {
              }
              frame True {
                n275 = Send Notification(notification=w667, notifier=w668) -> ()  [unwired: 1 in, 2 out]
              }
            }
          }
          frame "get_loop_iteration_terminal" {
            # "Returns the loops iteration terminal to be used for wiring."
            n276 = Variant To Data(error in=w679, type=T28 {"loop_id"=0, "Wait Notifier"=refnum, "wait for reply"=FALSE} ("get_loop_iteration_terminal Argument"), Variant=w676) -> (data=w670:T28, error out=w677:errorcluster)
            n277 = Unbundle By Name(w670) -> ("Wait Notifier"=w674:refnum<notifier>, "wait for reply"=w673:bool)  [unwired: 1 out]
            n278 = call "do get loop iteration terminal.vi"("error in (no error)"=w677, "get_loop_iteration_terminal Argument"=w670, "Data Cluster in"=w678) -> ("error out"=w671:errorcluster, "get_loop_iteration_terminal (Reply Payload)"=w672:T58, "Data Cluster out"=w669:T2)  [unwired: 6 in]
            n279 = case "DQMH_FIRE_NOTIFIER" shown="True" w673 {
              tunnel: w674 -> [_ w681]
              tunnel: w672 -> [_ w680]
              frame False {
              }
              frame True {
                n280 = Send Notification(notification=w680, notifier=w681) -> ()  [unwired: 1 in, 2 out]
              }
            }
          }
          frame "Read Config Data" {
            # "Reads the config data from the config file."
            n281 = call <vilib>:"Application Directory.vi"() -> ("Application Directory"=w691:path)
            n282 = Strip Path(path=w691) -> (stripped path=w690:path)  [unwired: 1 out]
            n283 = Build Path(base path=w690, name or relative path="config.json") -> (appended path=w688:path)
            n284 = Unbundle By Name(w685) -> ("Config Data"=w684:T3)
            n285 = Read from Text File(file (use dialog)=w688, error in=w693) -> (text=w686:string, error out=w692:errorcluster)  [unwired: 2 in, 2 out]
            n286 = Unflatten From JSON(JSON string=w686, type and defaults=w684, error in (no error)=w692) -> (value=w682:T3, error out=w687:errorcluster)  [unwired: 4 in]
            n287 = Bundle By Name(cluster=w685, "Config Data"=w682) -> (w683:T2)
          }
          frame "get_allowed_paths" {
            # "Returns the Directories that the Server can write files/folders to. If you try to write to other locations you will receive an error. If asked to save to a relative path, use this function to build the full path."
            n288 = Variant To Data(error in=w705, type=T30 {"Wait Notifier"=refnum, "wait for reply"=FALSE} ("get_allowed_paths Argument"), Variant=w704) -> (data=w702:T30, error out=w694:errorcluster)
            n289 = Unbundle By Name(w697) -> ("Config Data.Allowed Paths"=w696:string[])
            n290 = Unbundle By Name(w702) -> ("Wait Notifier"=w701:refnum<notifier>, "wait for reply"=w700:bool)
            n291 = for {
              tunnel: w696 -> [w708] mode=indexing
              tunnel: [w706] -> w695 mode=concatenating
              n292 = Format Into String(format string="\"%s\", ", w708) -> (resulting string=w706:string)  [unwired: 2 in, 1 out]
            }
            n293 = Bundle By Name(cluster=T54 {"Allowed Paths"="", "error"={"status"=FALSE, "code"=0, "source"=""}} ("get_allowed_paths (Reply Payload)"), "Allowed Paths"=w695, "error"=w694) -> (w699:T54)
            n294 = case "DQMH_FIRE_NOTIFIER" shown="True" w700 {
              tunnel: w701 -> [_ w710]
              tunnel: w699 -> [_ w709]
              frame False {
              }
              frame True {
                n295 = Send Notification(notification=w709, notifier=w710) -> ()  [unwired: 1 in, 2 out]
              }
            }
          }
          frame "create_project" {
            # "Creates a new Project at the specified location"
            n296 = Variant To Data(error in=w721, type=T31 {"File Path"="", "Wait Notifier"=refnum, "wait for reply"=FALSE} ("create_project Argument"), Variant=w718) -> (data=w711:T31, error out=w719:errorcluster)
            n297 = Unbundle By Name(w711) -> ("Wait Notifier"=w716:refnum<notifier>, "wait for reply"=w715:bool)
            n298 = call "Do create project.vi"("error in (no error)"=w719, "create_project Argument"=w711, "Data Cluster in"=w720) -> ("error out"=w713:errorcluster, "create_project (Reply Payload)"=w714:T59, "Data Cluster out"=w712:T2)  [unwired: 6 in]
            n299 = case "DQMH_FIRE_NOTIFIER" shown="True" w715 {
              tunnel: w716 -> [_ w723]
              tunnel: w714 -> [_ w722]
              frame False {
              }
              frame True {
                n300 = Send Notification(notification=w722, notifier=w723) -> ()  [unwired: 1 in, 2 out]
              }
            }
          }
          frame "Set Working Directory" {
            # "Sets the allowed directory for the AI. This function shall not be exposed to the LLM."
            n301 = Variant To Data(error in=w732, type=T32 {"Working Directory Folder Path"=[]} ("Set Working Directory Argument"), Variant=w729) -> (data=w727:T32, error out=w730:errorcluster)
            n302 = Unbundle By Name(w727) -> ("Working Directory Folder Path"=w725:path[])
            n303 = Path To String(path=w725) -> (string=w724:string[])
            n304 = Bundle By Name(cluster=w731, "Config Data.Allowed Paths"=w724) -> (w726:T2)
          }
          frame "---Copy This Frame---" {
            # "Duplicate this frame when creating new messages.  Change this comment in the duplicated frame to describe this message."
            n305 = Merge Errors(w735) -> (w734:errorcluster)
          }
          frame "---Exit and Error Handling---" {
            # "Separator - The following cases handle errors and exit messages."
          }
          frame "Simulate MHL Error" {
            # "#DQMH_HowTo The 'Simulate MHL Error' button  illustrates how the MHL handles errors. This event is instructional in nature and can be removed."
            # "Simulate an error occurring at the MHL"
            n306 = call "Module Name--constant.vi"() -> ("Module Name"=w739:string)  [unwired: 11 in]
            n307 = Format Into String(format string="Simulated error originating at Message Handling Loop in %s", w739) -> (resulting string=w740:string)  [unwired: 2 in, 1 out]
            n308 = call <vilib>:"Error Cluster From Error Code.vi"("show call chain? (False)"=TRUE, "error message (\"\")"=w740, "error code (0)"=5001) -> ("error out"=w744:errorcluster)  [unwired: 6 in]
            n309 = Merge Errors(w746, w744) -> (w745:errorcluster)
          }
          frame "Error" {
            # "#DQMH_CodeRecommended - If the module is running in standalone mode (External Launch = FALSE), this code will pop up an error dialog and call the 'Exit' message if an error occurs. Add more fine-grained error management here."
            # "Error - Check the error message data and respond accordingly. This message is sent by the \"Error Handler\" VIs at the end of each loop in this application."
            n310 = property on="Property Node" class="Module Admin"(reference=w749) -> ("Accessors:External Launch"=w748:bool)  [unwired: 1 in, 2 out]
            n311 = Variant To Data(error in=w757, type=errorcluster {"status"=FALSE, "code"=0, "source"=""} ("error constant"), Variant=w751) -> (data=w747:errorcluster, error out=w755:errorcluster)
            n312 = local write "error out"(w747) -> ()
            n313 = call "Error Reported.vi"("Error"=w747) -> ()  [unwired: 10 in, 1 out]
            n314 = case shown="False" w748 {
              tunnel: [w762 _] -> w754
              tunnel: w750 -> [w760 _]
              tunnel: w747 -> [w761 _]
              frame False {
                n315 = disable-structure shown="Default" {
                  disable-tunnel: w761 -> [w763 _]
                  frame condition #0 (active) {
                    # "If the module is running standalone, then pop up an error dialog and call the \"Exit\" message."
                    n316 = call <vilib>:"Simple Error Handler.vi"("error in (no error)"=w763) -> ()  [unwired: 4 in, 5 out]
                  }
                  frame condition #1 {
                    # "To prevent the Simple Error Handler VI from being loaded (e.g. when deploying to a Real-Time target), add the Conditional Disable Symbol \"DQMH_Disable_SEH\" to your project and set it to TRUE."
                  }
                }
                n317 = call-poly <vilib>:"Delacor_lib_QMH_Enqueue Message (poly).vi"("Priority Message? (F)"=TRUE, "Message"="Exit", "Message Queue in"=w760) -> ("error out"=w762:errorcluster)  [unwired: 7 in, 1 out]
              }
              frame True {
                # "If the module was launched externally, calling the Error Reported broadcast VI is the only action performed by the \"Error\" message. The module's caller can then process the error appropriately."
              }
            }
            n318 = Merge Errors(w755, w754) -> (w753:errorcluster)
          }
          frame "Exit" {
            w768 = 91  # 91: not all Exit messages will have an argument
            w770 = TRUE  # Stop the VI
            # "Release the message queue reference"
            # "#DQMH_CodeNeeded - Add any required cleanup code here."
            # "Exit - Exit the application."
            n319 = Variant To Data(error in=w778, type=T5 {"Origin"="", "Exit via Stop Module Req?"=FALSE, "Wait for Module to stop?"=FALSE} ("Stop Argument"), Variant=w769) -> (data=w766:T5, error out=w775:errorcluster)
            n320 = call <vilib>:"Clear Errors.vi"("error in (no error)"=w775, "specific error code to clear (0: all)"=w768) -> ("error out"=w777:errorcluster)  [unwired: 4 in, 1 out]
            n321 = control-ref of="This VI"() -> (w765:refnum<vi>)
            n322 = call-dynamic "Delacor_lib_QMH_Release Message Queue.vi"("error in"=w777, "Message Queue"=w772) -> ("error out"=w776:errorcluster)  [unwired: 9 in]
            n323 = call "Handle Exit.vi"("Stop Argument"=w766, "Admin in"=w764, "VI reference"=w765) -> ("error out"=w774:errorcluster)  [unwired: 7 in, 1 out]
            n324 = Merge Errors(w776, w774) -> (w773:errorcluster)
            n325 = call "Error Reported.vi"("Error"=w773) -> ()  [unwired: 10 in, 1 out]
          }
          frame Default {
            # "'Default' case only runs if there is a message that isn't defined in any of the other cases.  Output a programming error."
            n326 = call "Module Name--constant.vi"() -> ("Module Name"=w783:string)  [unwired: 11 in]
            n327 = Format Into String(format string="The invalid message string \"%s\" was received in the Message Handling Loop for module \"%s\".", w784, w783) -> (resulting string=w779:string)  [unwired: 2 in, 1 out]
            n328 = call <vilib>:"Error Cluster From Error Code.vi"("show call chain? (False)"=TRUE, "error message (\"\")"=w779, "error code (0)"=1) -> ("error out"=w786:errorcluster)  [unwired: 6 in]
            n329 = Merge Errors(w787, w786) -> (w788:errorcluster)
          }
        }
        n330 = call-dynamic "Delacor_lib_QMH_Error Handler - Message Handling Loop.vi"("error in"=w317, "Message Queue in"=w316) -> ("dup error in"=w318:errorcluster)  [unwired: 8 in, 1 out]
      }
    }
    frame Error {
      # "Synchronize Caller Events.vi will inform Start Module.vi that the module has launched and will let the code calling Start Module.vi register for broadcasts and would permit the caller receive the broadcast that an error occurred at launch time."
      n331 = call-dynamic "Delacor_lib_QMH_Release Message Queue.vi"("error in"=w796, "Message Queue"=w789) -> ("error out"=w795:errorcluster)  [unwired: 9 in]
      n332 = call "Synchronize Caller Events.vi"("Singleton Module Admin in"=w790) -> ("error out"=w797:errorcluster)  [unwired: 9 in, 1 out]
      n333 = call "Module Name--constant.vi"() -> ("Module Name"=w793:string)  [unwired: 11 in]
      n334 = Format Into String(format string="An error occurred during initialization. %s is no longer running.", w793) -> (resulting string=w791:string)  [unwired: 2 in, 1 out]
      n335 = Merge Errors(w795, w797) -> (w798:errorcluster)
      n336 = call "Error Reported.vi"("Additional Information"=w791, "Error"=w798) -> ()  [unwired: 9 in, 1 out]
    }
  }
  n337 = Merge Errors(w14, w17) -> (w13:errorcluster)
  n338 = call "Close Module.vi"("error in"=w13, "Module Admin in"=w8) -> ("error out"=w15:errorcluster, "External Launch"=w1:bool, "Module Admin out"=w2:refnum<class "Delacor_lib_QMH_Module Admin.lvclass">)  [unwired: 7 in]
  n339 = Unregister For Events(event registration refnum=w7, error in=w15) -> (error out=w12:errorcluster)
  "error out" <- w12
  n340 = case "External Launch?" shown="True" w1 {
    tunnel: w12 -> [_ w799]
    frame False {
    }
    frame True {
      n341 = case shown="No Error" w799 {
        frame No Error {
          n342 = invoke on="Invoke Node" class="VI" method="FP.Close"() -> ()  [unwired: 3 in, 3 out]
        }
        frame Error {
          n343 = disable-structure shown="Default" {
            frame condition #0 (active) {
              n344 = invoke class="VI" method="FP.Open"("Activate"=TRUE ("Activate?")) -> ()  [unwired: 4 in, 5 out]
            }
            frame condition #1 {
              # "Don't show panel on error if running inside a built EXE."
            }
          }
        }
      }
    }
  }
  n345 = local write "Module Admin"(w2) -> ()
